vi "Main.vi"() -> ()   [LabVIEW 2017]
uses:
  type defs/action buttons.ctl
  type defs/mode buttons.ctl
  <vilib>/vision/Pattern Matching.llb/IMAQ GM Match Report.ctl
  type defs/states.ctl
  type defs/data.ctl
  <vilib>/vision/Image Controls.llb/IMAQ Image.ctl
  <vilib>/myRIO/Common/Instrument Driver Framework/myRIO v1.0/Encoder/typedefs/Encoder Signal Mode.ctl
  <vilib>/myRIO/Instrument Drivers/Onboard IO/PWM/typedefs/PWM Reference.ctl
  <vilib>/myRIO/Common/Instrument Driver Framework/Utilities/typedefs/myRIO Generic Hardware Reference.ctl
  <vilib>/myRIO/Common/Instrument Driver Framework/Utilities/typedefs/Hardware Version Enum.ctl
  <vilib>/myRIO/Common/Instrument Driver Framework/Utilities/typedefs/myRIO v1.0 Reference.ctl
  <vilib>/myRIO/Common/Instrument Driver Framework/Utilities/typedefs/Generic FPGA Reference.ctl
  <vilib>/myRIO/Common/Instrument Driver Framework/myRIO v1.0/PWM/typedefs/PWM Channels Enum.ctl
  <vilib>/myRIO/Instrument Drivers/Onboard IO/PWM/typedefs/PWM Configuration.ctl
  <vilib>/userdefined/High Color/nirio_resource_hc.ctl
  <vilib>/myRIO/Instrument Drivers/Onboard IO/DIO/typedefs/DIO Reference.ctl
  <vilib>/myRIO/Common/Instrument Driver Framework/myRIO v1.0/DIO/typedefs/DIO Channels List.ctl
  <vilib>/myRIO/Common/Instrument Driver Framework/myRIO v1.0/DIO/typedefs/DIO Channels Enum.ctl
  type defs/task.ctl
  <vilib>/myRIO/Common/Instrument Driver Framework/Utilities/vis/Is FPGA Ref Available.vi
  <vilib>/myRIO/Common/Instrument Driver Framework/myRIO v1.0/PWM/vis/myRIO v1.1 Open PWM.vi
  <vilib>/myRIO/Common/Instrument Driver Framework/myRIO v1.0/DIO/vis/myRIO v1.1 Open DIO.vi
  <vilib>/myRIO/Instrument Drivers/Onboard IO/DIO/vis/Write.vi
  <vilib>/myRIO/Common/Instrument Driver Framework/Utilities/vis/Validate Channels.vi
  <vilib>/myRIO/Common/Instrument Driver Framework/myRIO v1.0/PWM/vis/myRIO v1.0 Reserve PWM.vi
  <vilib>/myRIO/Common/Instrument Driver Framework/myRIO v1.0/DIO/vis/myRIO v1.0 Reserve DIO.vi
  <vilib>/myRIO/Common/Instrument Driver Framework/myRIO v1.0/Encoder/vis/myRIO v1.0 Close Encoder.vi
  <vilib>/myRIO/Common/Instrument Driver Framework/myRIO v1.0/PWM/vis/myRIO v1.0 Close PWM.vi
  <vilib>/myRIO/Common/Instrument Driver Framework/myRIO v1.0/UART/vis/myRIO v1.0 Close UART.vi
  <vilib>/myRIO/Common/Instrument Driver Framework/myRIO v1.0/PWM/vis/myRIO v1.0 Build MUX Configuration PWM.vi
  <vilib>/myRIO/Common/Instrument Driver Framework/myRIO v1.0/Resource Manager/vis/myRIO v1.0 Reserve Channel List.vi
  <vilib>/myRIO/Common/Instrument Driver Framework/myRIO v1.0/DIO/vis/myRIO v1.0 Build MUX Configuration DIO.vi
  <vilib>/myRIO/Common/Instrument Driver Framework/myRIO v1.0/Encoder/vis/myRIO v1.0 Unreserve Encoder.vi
  <vilib>/myRIO/Common/Instrument Driver Framework/myRIO v1.0/PWM/vis/myRIO v1.0 Unreserve PWM.vi
  <vilib>/myRIO/Common/Instrument Driver Framework/myRIO v1.0/Resource Manager/vis/myRIO v1.0 Create Configuration List.vi
  <vilib>/myRIO/Common/Instrument Driver Framework/myRIO v1.0/Resource Manager/vis/myRIO v1.0 Reserve Channel.vi
  <vilib>/myRIO/Common/Instrument Driver Framework/myRIO v1.0/Resource Manager/vis/myRIO v1.0 Unreserve Channel.vi
  <vilib>/myRIO/Common/Instrument Driver Framework/myRIO v1.0/Encoder/vis/myRIO v1.0 Build MUX Configuration Encoder.vi
  <vilib>/myRIO/Common/Instrument Driver Framework/myRIO v1.0/Resource Manager/vis/myRIO v1.0 Unreserve Channel List.vi
  <vilib>/myRIO/Common/Instrument Driver Framework/myRIO v1.0/Resource Manager/vis/myRIO v1.0 Build Mutex Name.vi
  <vilib>/Utility/VariantDataType/GetNumericInfo.vi
  <vilib>/Utility/error.llb/Error Cluster From Error Code.vi
  <vilib>/myRIO/Common/Instrument Driver Framework/myRIO v1.0/myRIO v1.1 Open.vi
  <vilib>/myRIO/Common/Instrument Driver Framework/Utilities/vis/IO Manager.vi
  <vilib>/myRIO/Common/Instrument Driver Framework/Utilities/vis/Configuration Manager.vi
  <vilib>/myRIO/Common/Instrument Driver Framework/myRIO v1.0/Resource Manager/vis/myRIO v1.0 Configure IO.vi
  <vilib>/myRIO/Common/Instrument Driver Framework/myRIO v1.0/myRIO v1.0 Close.vi
  <vilib>/myRIO/Common/Instrument Driver Framework/myRIO v1.0/Encoder/vis/myRIO v1.0 Reset Encoder.vi
  <vilib>/myRIO/Common/Instrument Driver Framework/myRIO v1.0/PWM/vis/myRIO v1.0 Write PWM.vi
  <vilib>/myRIO/Common/Instrument Driver Framework/myRIO v1.0/Encoder/vis/myRIO v1.0 Read Encoder.vi
  <vilib>/myRIO/Common/Instrument Driver Framework/myRIO v1.0/DIO/vis/myRIO v1.0 Write DIO.vi
  <vilib>/myRIO/Common/Instrument Driver Framework/myRIO v1.0/DIO/vis/myRIO v1.0 Read DIO.vi
  <vilib>/myRIO/Common/Instrument Driver Framework/myRIO v1.0/PWM/vis/myRIO v1.0 Shutdown PWM.vi
  <vilib>/myRIO/Common/Instrument Driver Framework/myRIO v1.0/Encoder/vis/myRIO v1.0 Shutdown Encoder.vi
  <vilib>/myRIO/Common/Instrument Driver Framework/Utilities/vis/FPGA Ref Manager.vi
  <vilib>/myRIO/Common/Instrument Driver Framework/myRIO v1.0/myRIO v1.0 Reset FPGA.vi
  <vilib>/myRIO/Common/Instrument Driver Framework/myRIO v1.0/IRQ/vis/myRIO v1.0 IRQ Info FGV.vi
  <vilib>/myRIO/Common/Instrument Driver Framework/myRIO v1.0/IRQ/vis/myRIO v1.0 Timer IRQ Info FGV.vi
  <vilib>/myRIO/Common/Instrument Driver Framework/myRIO v1.0/IRQ/vis/myRIO v1.0 ISR Agent.vi
  <vilib>/myRIO/Instrument Drivers/Onboard IO/I2C/typedefs/I2C Reference.ctl
  <vilib>/myRIO/Common/Instrument Driver Framework/myRIO v1.0/I2C/typedefs/I2C Channels Enum.ctl
  <vilib>/myRIO/Instrument Drivers/Onboard IO/I2C/typedefs/I2C Configuration.ctl
  <vilib>/myRIO/Instrument Drivers/Onboard IO/I2C/typedefs/I2C Transfer Rate.ctl
  <vilib>/myRIO/Express VI/Onboard IO/PWM/PWM Express VI.xnode
  <vilib>/myRIO/Instrument Drivers/Onboard IO/PWM/vis/myRIO PWM Open.xnode
  <vilib>/myRIO/Express VI/Onboard IO/DO/DO Express VI.xnode
  <vilib>/myRIO/Instrument Drivers/Onboard IO/DIO/vis/myRIO DIO Open.xnode
  <vilib>/myRIO/Express VI/Onboard Devices/LED/LED Express VI.xnode
  <vilib>/myRIO/Express VI/Onboard Devices/Button/Button Express VI.xnode
  <vilib>/myRIO/Instrument Drivers/Onboard IO/DIO/DIO.lvlib
  <vilib>/myRIO/Instrument Drivers/Onboard IO/PWM/PWM.lvlib
  <vilib>/myRIO/Instrument Drivers/Utilities/Utilities.lvlib
  <vilib>/vision/NI_Vision_Development_Module.lvlib
  <vilib>/myRIO/Instrument Drivers/Onboard IO/I2C/I2C.lvlib
  <vilib>/myRIO/Instrument Drivers/Onboard IO/I2C/vis/myRIO I2C Open.xnode
  <vilib>/myRIO/Common/Instrument Driver Framework/myRIO v1.0/I2C/vis/myRIO v1.1 Open I2C.vi
  <vilib>/myRIO/Instrument Drivers/Onboard IO/Encoder/Encoder.lvlib
panel:
  out "FT_G_enc":i32[](array[numeric])
  out "FT_M_enc":i32[](array[numeric])
  out "FT_Right_enc":i32[](array[numeric])
  out "FT_Left_enc":i32[](array[numeric])
  out "FT_Angles":dbl[](array[numeric])
  out "Dots of States":i32[][](array[numeric])
  in  "States in total":i32
  in  "(auto) States":T1(ring)
  out "R_enc_value":i32
  in  "Reset R_enc":bool
  out "L_enc_value":i32
  in  "Reset L_enc":bool
  out "G_enc":i32[](array[numeric])
  out "M_enc":i32[](array[numeric])
  out "Right_enc":i32[](array[numeric])
  out "Left_enc":i32[](array[numeric])
  out "Angles":dbl[](array[numeric])
  in  "Dots in total":i32
  in  "CurDot":T2(ring)
  out "balls to analyze":i32[](array[numeric])
  out "(auto) balls counter":i32
  out "distance to the side":u32
  out "value Z 2":ext
  out "value Z":ext
  in  ",ctl num":i32
  in  ".Task":enum16{"Def", "<mod>[P]+tnl ", "(auto)"}(ring)
  in  "_Timer":u32=1
  out "Pattern classes":i32[](array[numeric])
  in  "5":i32
  in  "4":i32
  in  "3":i32
  in  "1":i32
  in  "2":i32
  out "5":bool
  out "4":bool
  out "3":bool
  out "2":bool
  out "1":bool
  out "Color classes":i32[](array[numeric])
  in  "Next step":bool
  in  "ball = pattern?":bool
  out "error out":errorcluster
  in  "Tab Control":enum32{"Motors", "Ball", "Pattern", "Camera"}(tab)
  in  "Left+":bool
  in  "Left-":bool
  in  "Right+":bool
  in  "Right-":bool
  in  "G-":bool
  in  "G+":bool
  in  "M+":bool
  in  "M-":bool
  in  "M_PWM":dbl=0.5
  in  "L_PWM":dbl=0.5
  in  "R_PWM":dbl=0.5
  in  "Reset M_enc":bool
  out "M_enc_value":i32
  in  "Reset G_enc":bool
  out "G_enc_value":i32
  in  "G_PWM":dbl=0.5
  in  "M_UB_Align":i32=-800
  in  "G_UB_Align":i32
  in  "M_UB_grab":i32=-800
  in  "G_UB_grab":i32=-500
  in  "Manip state":enum16{"Align", "Grab", "Release"}(ring)
  in  "Balls to remember":i32
  out "Circles Calibrated (Shape Detection 1)":T3(array[cluster]) {"Position"."Y" format="%.2f"; "Position"."X" format="%.2f"}
  out "Number of Matches (Shape Detection 1)":i32
  out "Color":i32
  in  "Align X - t, Y - f":bool
  out "CircleRadius":dbl
  in  "defX":dbl=150.0
  in  "Range":dbl=40.0
  in  "defY":dbl=170.0
  out "X is in range":bool
  out "Y is in range":bool
  out "curX":dbl
  out "curY":dbl
  out "y1 (circle)":i32
  out "x1 (circle)":i32
  out "x0 (circle)":i32
  out "y0 (circle)":i32
  in  "divider (circle)":dbl=1.0
  in  "ROI Descriptor COLOR":T4={"Global Rectangle"=[86, 71, 180, 164], "Contours"=[{"ID"=enum."External", "Type"=3, "Coordinates"=[86, 71, 180, 164]}]} {"Contours"."Type" items=["No Selection", "Point", "Line", "Rectangle", "Oval", "Polygon", "Freehand Region", "Annulus", "Unused2", "Unused3", "Broken Line", "Freehand Line", "Rotated Rectangle"]}
  in  "align accuracy":u32=100
  in  "Ball number":i32=1
  out "ball match":bool
  in  "Range(p)":sgl=10.0
  in  "defX(p)":sgl=320.0
  out "Pattern":i32
  out "y0":i32
  out "x0":i32
  out "x1":i32
  out "y1":i32
  out "Number of Matches (Geometric Matching 1)":i32
  out "Calibrated Matches (Geometric Matching 1)":T5[](array[typedef]) {"Correlation Score" format="%.2f"; "Target Template Curve Score" format="%.2f"; "Template Target Curve Score" format="%.2f"; "Bounding Box"."y" format="%.2f"; "Bounding Box"."x" format="%.2f"; "Position"."y" format="%.2f"; "Position"."x" format="%.2f"; "Score" format="%.2f"; "Scale" format="%.2f"; "Angle" format="%.2f"; "Occlusion %" format="%.2f"}
  out "Scale":sgl
  in  "divider (pattern)":sgl=1.0
  out "curX(p)":sgl
  out "In Range? (p)":bool
  in  "align accuracy (p)":u32=100
  in  "pattern number":i32=1
  in  "patterns to remember":i32=3
  out "pattern match":bool
  in  "M duty cycle [P]":dbl=533.0 format="%#_13g"
  in  "S duty cycle [P]":dbl=990.0 format="%#_13g"
  in  "S duty cycle [B]":dbl=990.0 format="%#_13g"
  in  "M duty cycle [B]":dbl=533.0 format="%#_13g"
  in  "S duty cycle [F]":dbl=620.0 format="%#_13g"
  in  "M duty cycle [F]":dbl=506.0 format="%#_13g"
  in  "Angle for pattern (degrees)":sgl=90.0 format="%.2f"
  out "rotate":bool=TRUE
  in  "PWM channel (m)":tag="B/PWM2"
  in  "[cur] duty cycle [%] (m)":dbl
  in  "PWM channel (s)":tag="A/PWM2"
  in  "[cur] duty cycle [%] (s)":dbl
  in  "Camera state":enum16{"Fwd", "Pattern", "Ball"}(ring)
  in  "Angle for Align (degrees)":sgl=2.0 format="%.2f"
  in  "mode buttons":T6
  out "image display":T7(plugin-control)
  in  "action buttons":T8
  in  "Stop":bool
  # "Machine\nVision\nApp"
  # "less = slower"
  # "less = slower"
  # "0 - 640x480"
  # "5 - 1280x720"
  # "30 - 320x240"
  # "35 - 800x600"
  # "40 - 176x144"
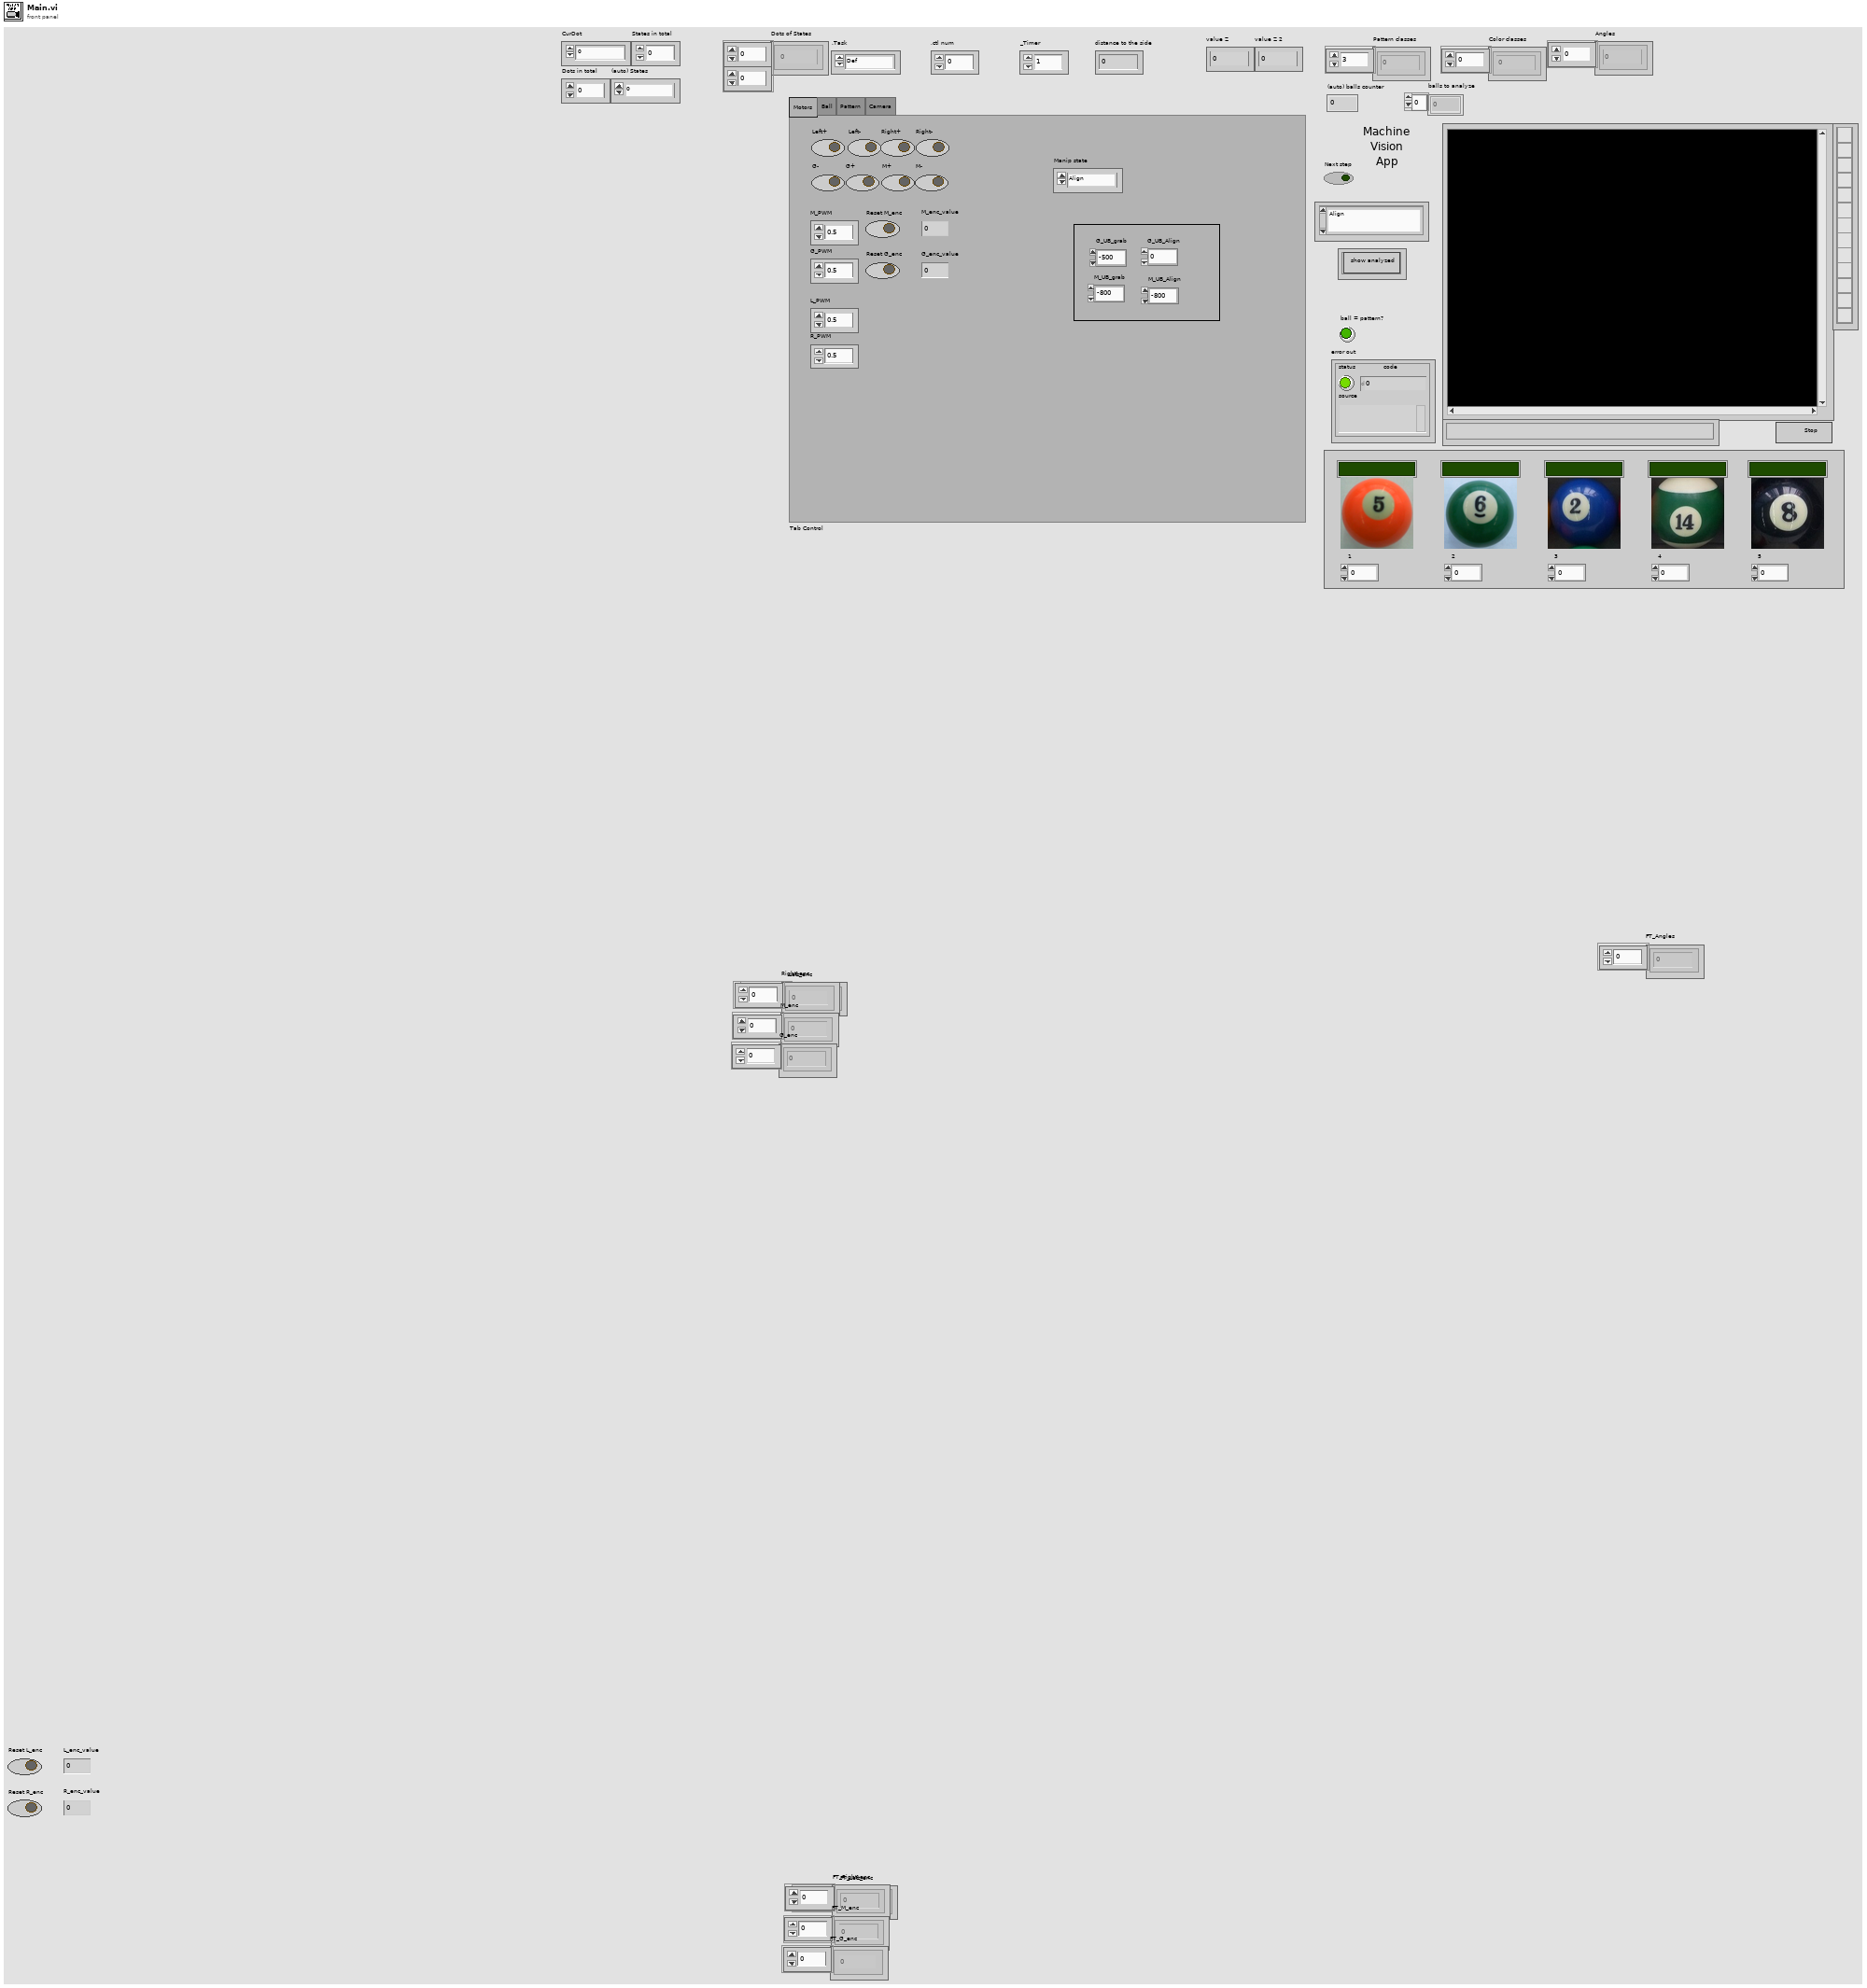
[diagram p1: front panel]
types:
  T1 = enum16{"0", "1", "2", "3", "4", "5", "6", "7", "8", "9", "10"}
  T2 = enum16{"0", "1", "2", "3", "4", "5", "6", "7", "8", "9", "10", "11", "12", "13", "14", "15", "16", "17", "18", "19", "20", "21", "22", "23", "24", "25", "26", "27", "28", "29", "30", "31", "32", "33", "34", "35"}
  T3 = cluster{"Position":cluster{"X":sgl, "Y":sgl}, "Radius":dbl, "Score":dbl}[]
  T4 = cluster{"Global Rectangle":i32[], "Contours":cluster{"ID":enum32{"External", "Internal"}, "Type":u32, "Coordinates":i32[]}[]}
  T5 = typedef "IMAQ GM Match Report.ctl" = cluster{"Position":cluster{"x":sgl, "y":sgl}, "Angle":sgl, "Scale":sgl, "Score":sgl, "Bounding Box":cluster{"x":sgl, "y":sgl}[], "Contrast Reversed":bool, "Occlusion %":sgl, "Template Target Curve Score":sgl, "Target Template Curve Score":sgl, "Correlation Score":sgl}
  T6 = typedef "mode buttons.ctl" = cluster{"show analyzed":bool}
  T7 = typedef "IMAQ Image.ctl" = refnum<image>
  T8 = typedef "action buttons.ctl" = cluster{"Shape - t, Color - f":enum16{"Align", "(pattern) Align", "Pattern", "(mod) pattern", "<mod>[P] remembering", "<mod>[P] go through tunnel", "<mod>[P] comparing", "(mod) ball", "Ball", "Other", "Clear", "navx", "(auto) Balls Analyze", "Joystick control"}}
  T9 = typedef "Encoder Signal Mode.ctl" = enum16{"Quadrature phase signal", "Step and direction signal"}
  T10 = typedef "data.ctl" = cluster{"Shape - t, Color - f":bool, "qsm":cluster{"Webcam image ref":T7, "Analyzed image ref":T7, "Stop webcam":bool}, " image ref":T7, "number img":i32, "ROI Descriptor (Image Mask 1)":cluster{"Global Rectangle":i32[], "Contours":cluster{"ID":enum32{"External", "Internal"}, "Type":u32, "Coordinates":i32[]}[]}, "Pattern class":i32, "Color class":i32, "Color classes":i32[], "Pattern classes":i32[]}
  T11 = typedef "states.ctl" = enum16{"(qsm) schedule", "(qsm) initialize", "(qsm) release", "(qsm) clean up", "(qsm) shutdown", "(myRIO) initialize", "(myRIO) clean up", "(myRIO) update ports", "Setup get", "(image) get", "(image) show", "(ball) Shape detection", "(ball) Calc ball indx", "(ball) Calculate ROI", "(ball) Analyze color", "(ball) Align", "(ball) Wait", "(ball) Grab", "(pattern) Find Square", "(pattern) Calculate ROI", "(pattern) Calc pattern indx", "Compare", "(pattern) Analyze pattern", "(pattern) Align", "(pattern) Wait", "(pattern) states control", "navx", "stop motors", "(joystick) Joystick control", "_Timer", "Setup manipulator", "(auto) Count balls", "(auto) Analyze balls", "(auto) Dot Controller", "Wait for button"}
  T12 = typedef "Encoder.lvlib/Encoder Reference.ctl" = cluster{"myRIO Reference":T13, "Encoder Channels Enum":T17}
  T13 = typedef "myRIO Generic Hardware Reference.ctl" = cluster{"myRIO Model":T14, "myRIO Hardware Reference":T15}
  T14 = typedef "Hardware Version Enum.ctl" = enum16{"Unknown", "myRIO-1900", "myRIO-1950", "roboRIO", "NI ELVIS RIO CM"}
  T15 = typedef "myRIO v1.0 Reference.ctl" = cluster{"Generic FPGA Reference":T16, "Allow multiple opens":bool}
  T16 = typedef "Generic FPGA Reference.ctl" = refnum<k20>
  T17 = typedef "Encoder Channels Enum.ctl" = enum16{"Not Connected", "C/ENC0", "C/ENC1", "A/ENC", "B/ENC", "DIO/ENC0", "DIO/ENC1", "DIO/ENC2", "DIO/ENC3", "DIO/ENC4"}
  T18 = typedef "PWM.lvlib/PWM Reference.ctl" = cluster{"myRIO Reference":T13, "PWM Channels Enum":T19, "PWM Configuration":T20}
  T19 = typedef "PWM Channels Enum.ctl" = enum16{"Not Connected", "C/PWM0", "C/PWM1", "A/PWM0", "A/PWM1", "A/PWM2", "B/PWM0", "B/PWM1", "B/PWM2", "PWM/PWM0", "PWM/PWM1", "PWM/PWM2", "PWM/PWM3", "PWM/PWM4", "PWM/PWM5", "PWM/PWM6", "PWM/PWM7", "PWM/PWM8", "PWM/PWM9"}
  T20 = typedef "PWM.lvlib/PWM Configuration.ctl" = cluster{"Frequency":dbl, "Duty Cycle":dbl}
  T21 = typedef "nirio_resource_hc.ctl" = tag
  T22 = typedef "I2C.lvlib/I2C Reference.ctl" = cluster{"myRIO Reference":T13, "I2C Channels Enum":T23, "I2C Configuration":T24}
  T23 = typedef "I2C Channels Enum.ctl" = enum16{"Not Connected", "A/I2C", "B/I2C", "I2C/I2C"}
  T24 = typedef "I2C.lvlib/I2C Configuration.ctl" = cluster{"I2C Transfer Rate":T25}
  T25 = typedef "I2C.lvlib/I2C Transfer Rate.ctl" = enum16{"Standard mode (100 kbps)", "Fast mode (400 kbps)"}
  T26 = typedef "DIO.lvlib/DIO Reference.ctl" = cluster{"myRIO Reference":T13, "DIO Channels List":T27}
  T27 = typedef "DIO Channels List.ctl" = T28[]
  T28 = typedef "DIO Channels Enum.ctl" = enum16{"Not Connected", "C/DIO0", "C/DIO1", "C/DIO2", "C/DIO3", "C/DIO4", "C/DIO5", "C/DIO6", "C/DIO7", "A/DIO0", "A/DIO1", "A/DIO2", "A/DIO3", "A/DIO4", "A/DIO5", "A/DIO6", "A/DIO7", "A/DIO8", "A/DIO9", "A/DIO10", "A/DIO11", "A/DIO12", "A/DIO13", "A/DIO14", "A/DIO15", "B/DIO0", "B/DIO1", "B/DIO2", "B/DIO3", "B/DIO4", "B/DIO5", "B/DIO6", "B/DIO7", "B/DIO8", "B/DIO9", "B/DIO10", "B/DIO11", "B/DIO12", "B/DIO13", "B/DIO14", "B/DIO15", "LED0", "LED1", "LED2", "LED3", "Button0", "DIO/DIO0", "DIO/DIO1", "DIO/DIO2", "DIO/DIO3", "DIO/DIO4", "DIO/DIO5", "DIO/DIO6", "DIO/DIO7", "DIO/DIO8", "DIO/DIO9", "SPI/CS0", "SPI/CS1", "SPI/CS2", "SPI/CS3", "LED RADIO (Green)", "LED RADIO (Red)", "LED COMM (Green)", "LED COMM (Red)", "LED MODE (Green)", "LED MODE (Red)"}
  T29 = enum16{"Align", "(pattern) Align", "Pattern", "(mod) pattern", "(mod) ball", "Ball", "Other", "Clear", "Joystick control"}
  T30 = enum16{"Align", "(pattern) Align", "Pattern", "(mod) pattern", "<mod>[P] remembering", "<mod>[P] go through tunnel", "<mod>[P] comparing", "(mod) ball", "Ball", "Other", "Clear", "navx", "(auto) Balls Analyze", "Joystick control"}
  T31 = enum16{"Align", "(pattern) Align", "Pattern", "(mod) pattern", "<mod>[P] remembering", "<mod>[P] go through tunnel", "<mod>[P] comparing", "(mod) ball", "Ball", "Other", "Clear", "Joystick control"}
  T32 = enum16{"Align", "(pattern) Align", "Pattern", "(mod) pattern", "<mod>[P]+move", "(mod) ball", "Ball", "Other", "Clear", "Joystick control"}
  T33 = typedef "task.ctl" = T11[]
  T34 = typedef "Image Type" = u32
  T35 = cluster{"Position":cluster{"X":sgl, "Y":sgl}, "Radius":dbl, "Score":dbl}
  T36 = cluster{"ID":enum32{"External", "Internal"}, "Type":u32, "Coordinates":i32[]}[]
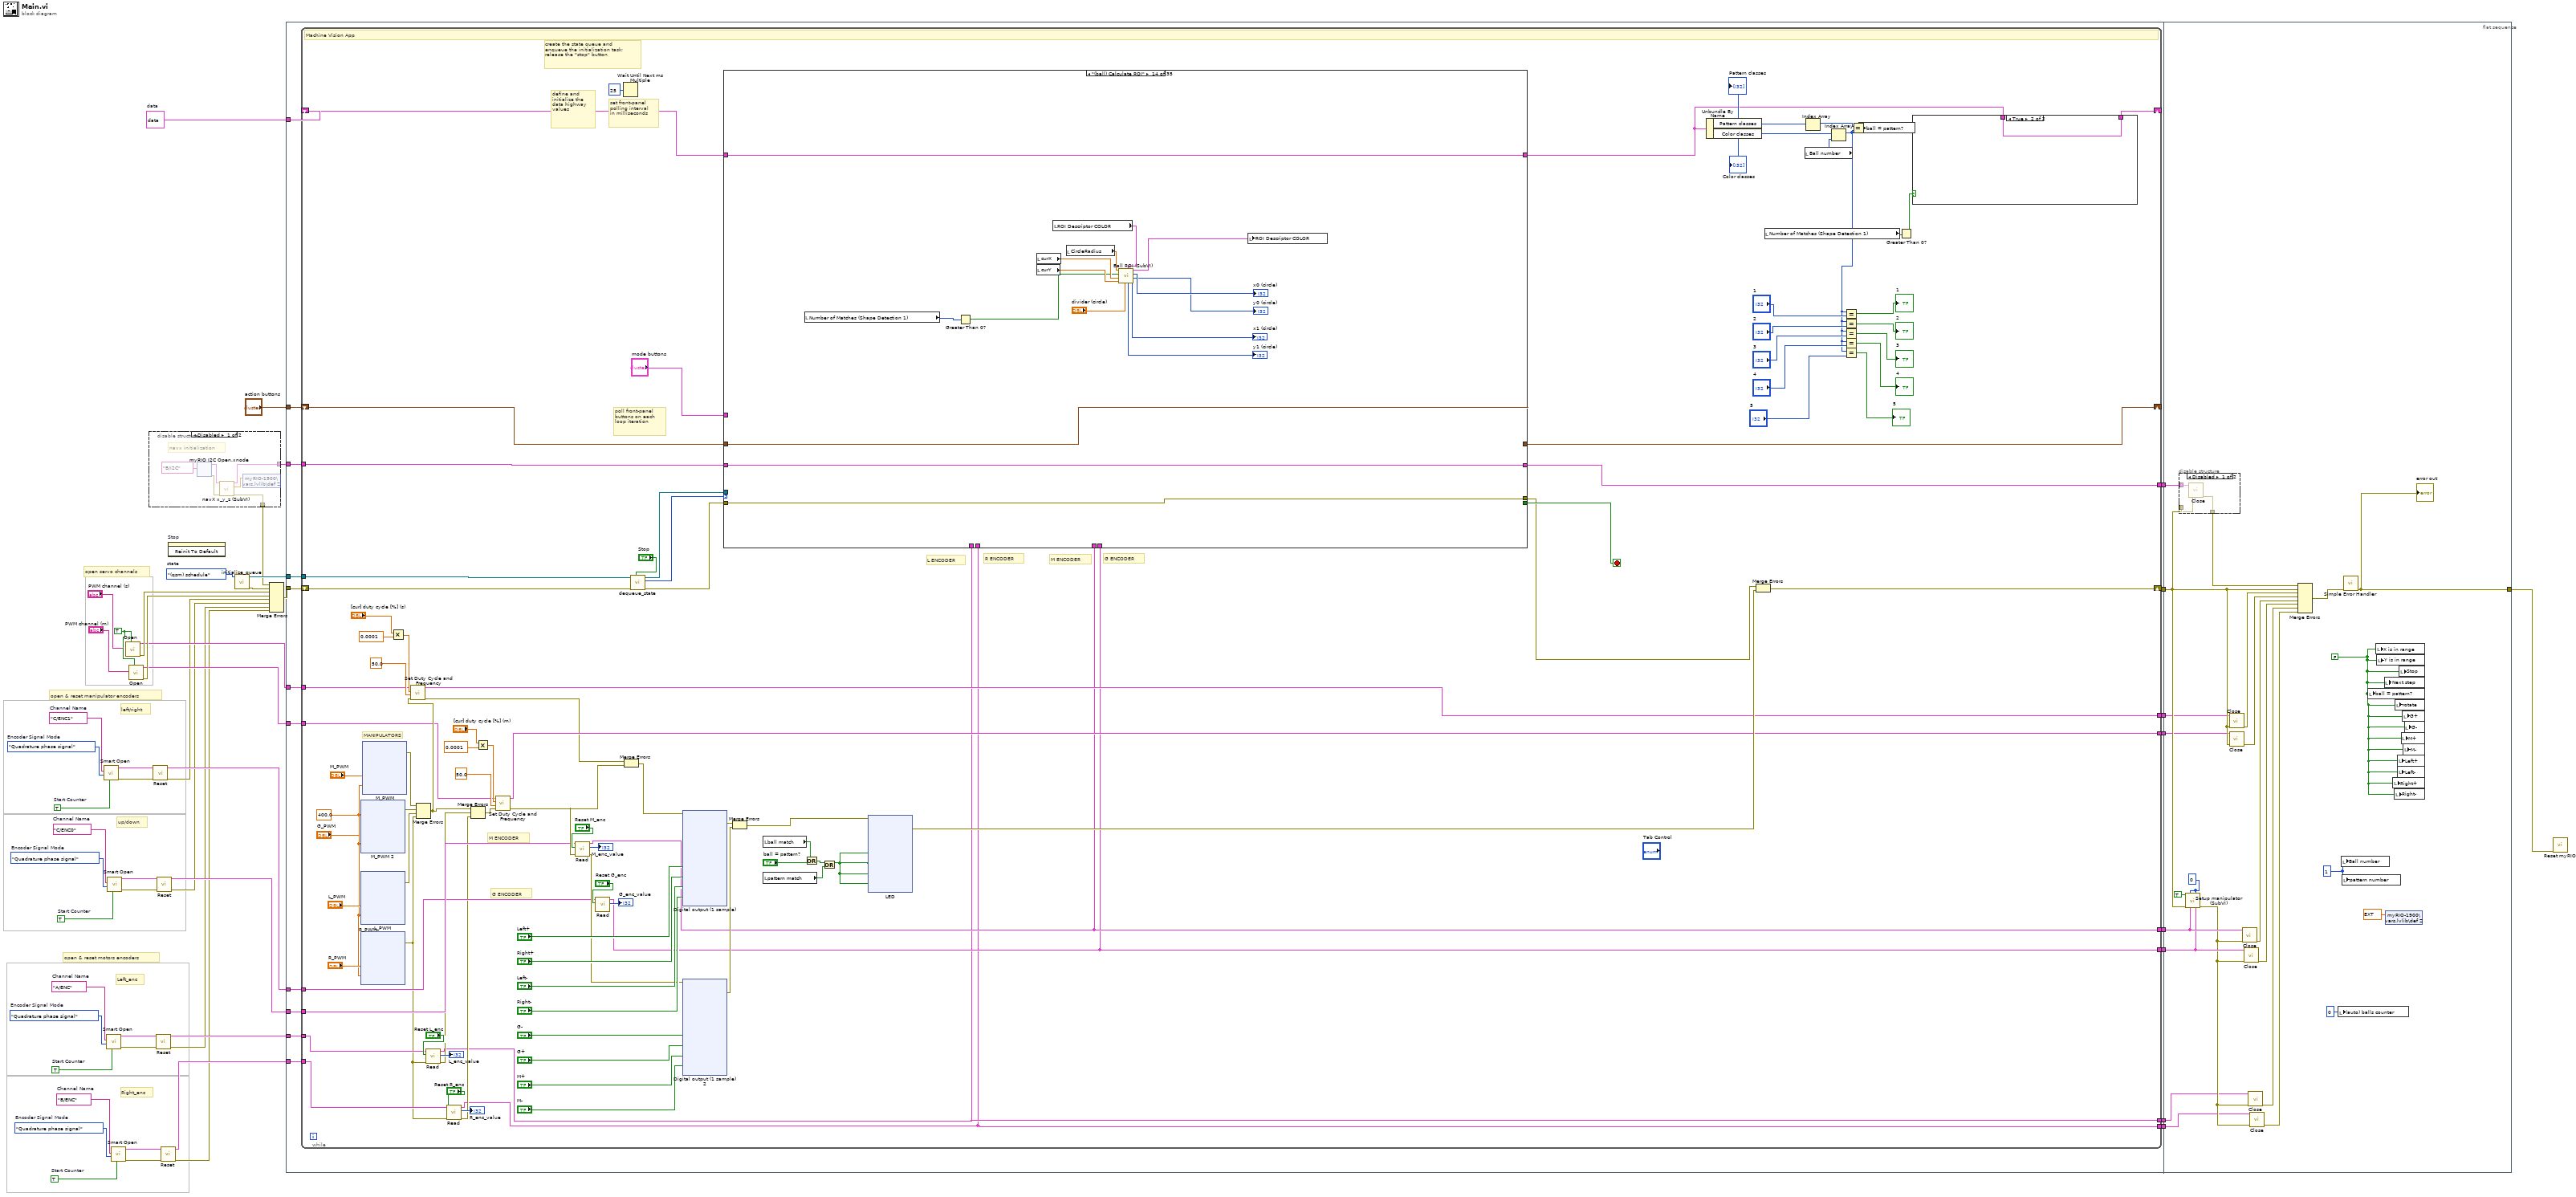
[diagram p0: block diagram]
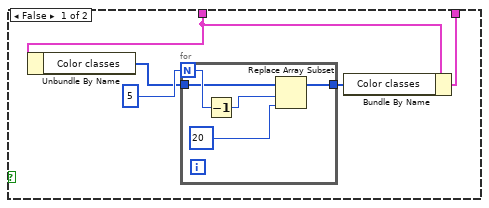
[diagram p3: hidden frame]
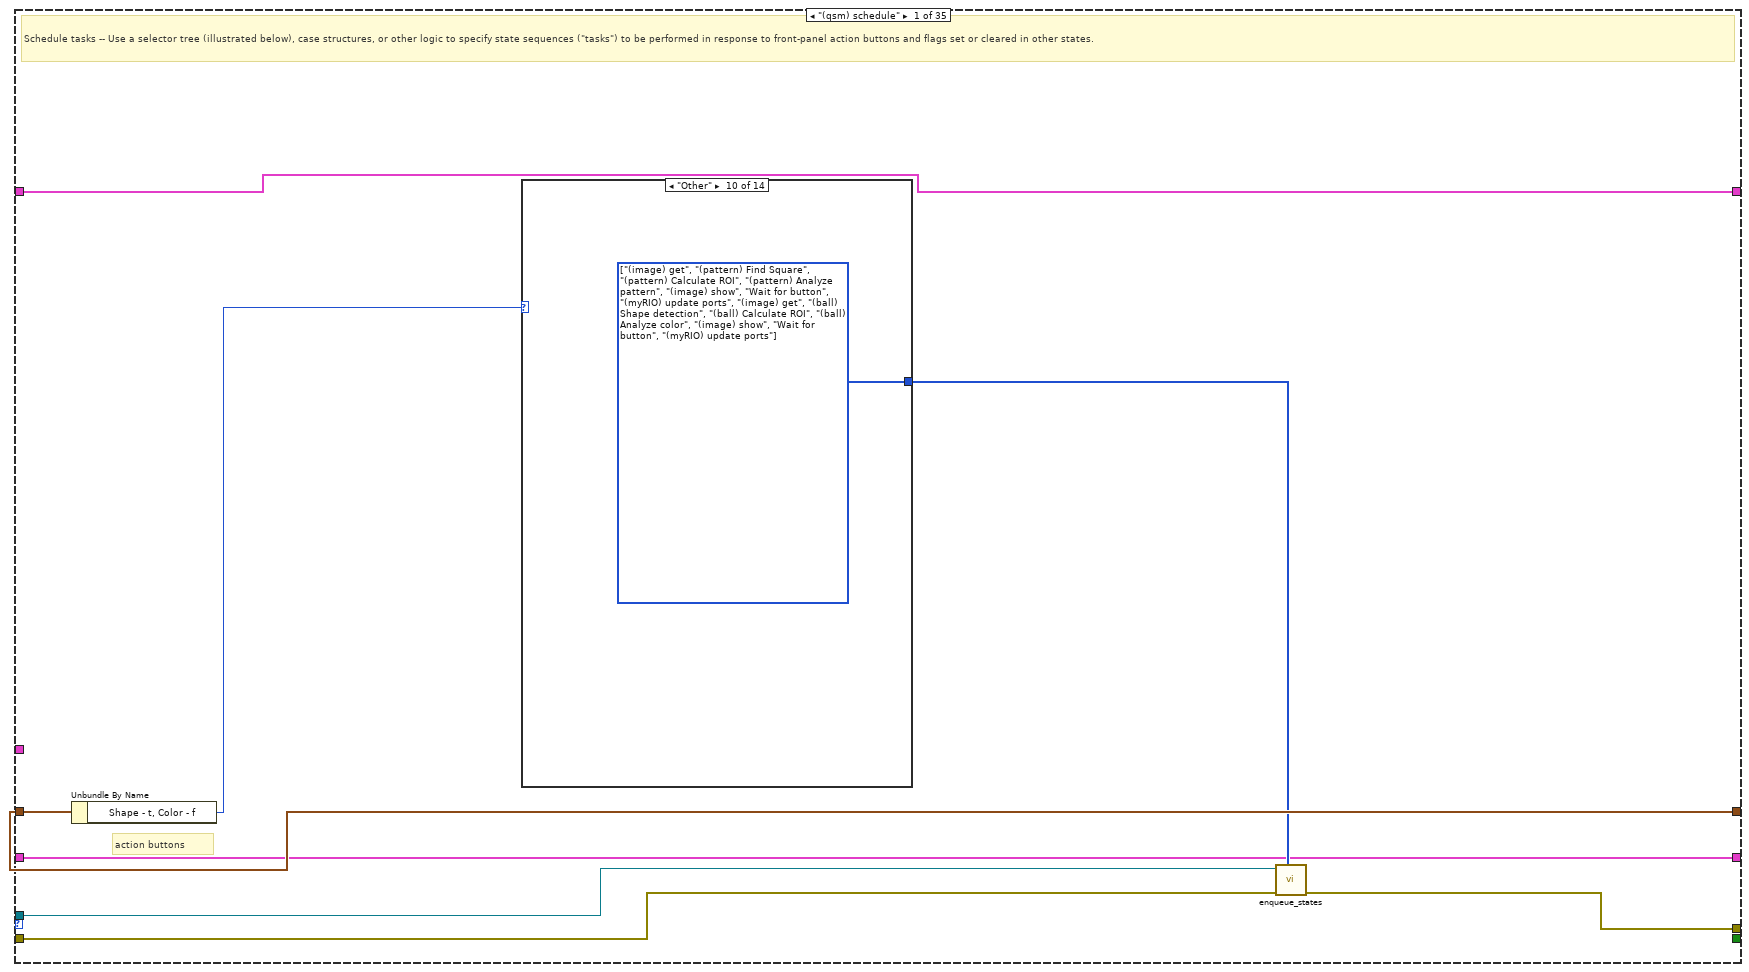
[diagram p4: hidden frame]
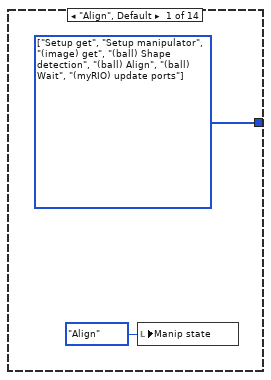
[diagram p5: hidden frame]
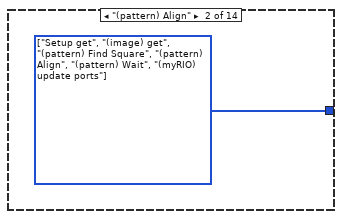
[diagram p6: hidden frame]
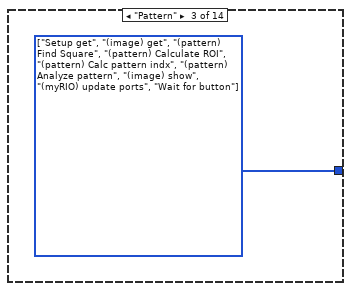
[diagram p7: hidden frame]
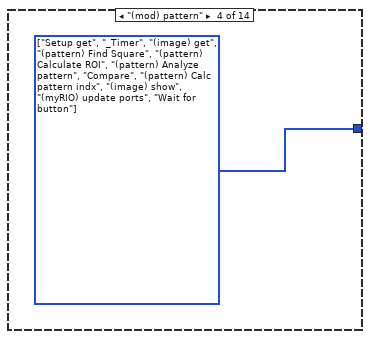
[diagram p8: hidden frame]
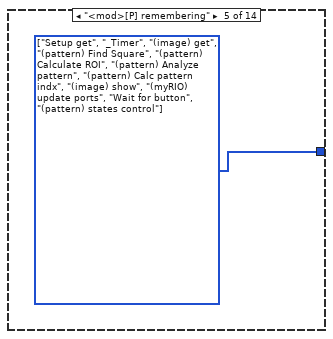
[diagram p9: hidden frame]
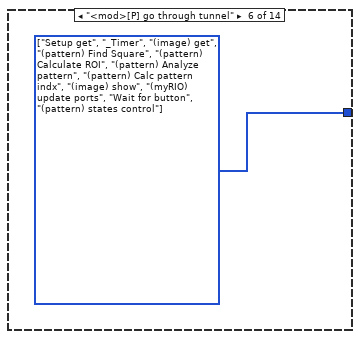
[diagram p10: hidden frame]
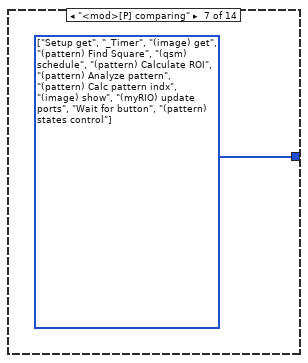
[diagram p11: hidden frame]
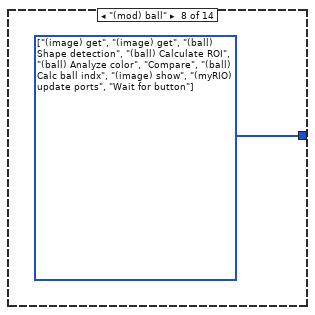
[diagram p12: hidden frame]
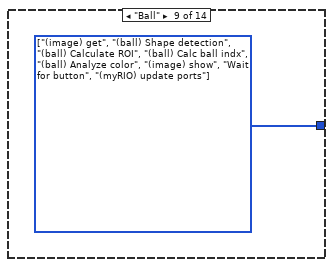
[diagram p13: hidden frame]
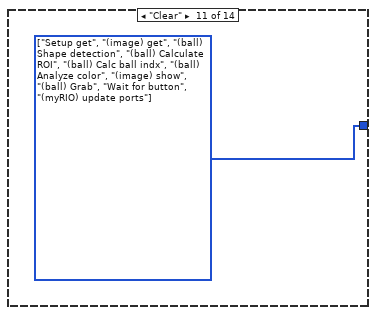
[diagram p14: hidden frame]
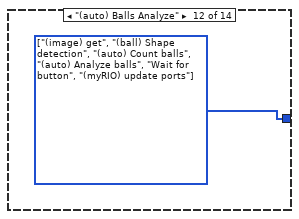
[diagram p15: hidden frame]
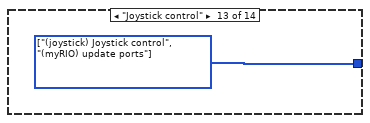
[diagram p16: hidden frame]
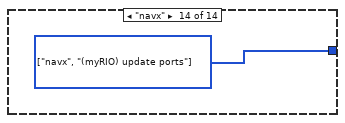
[diagram p17: hidden frame]
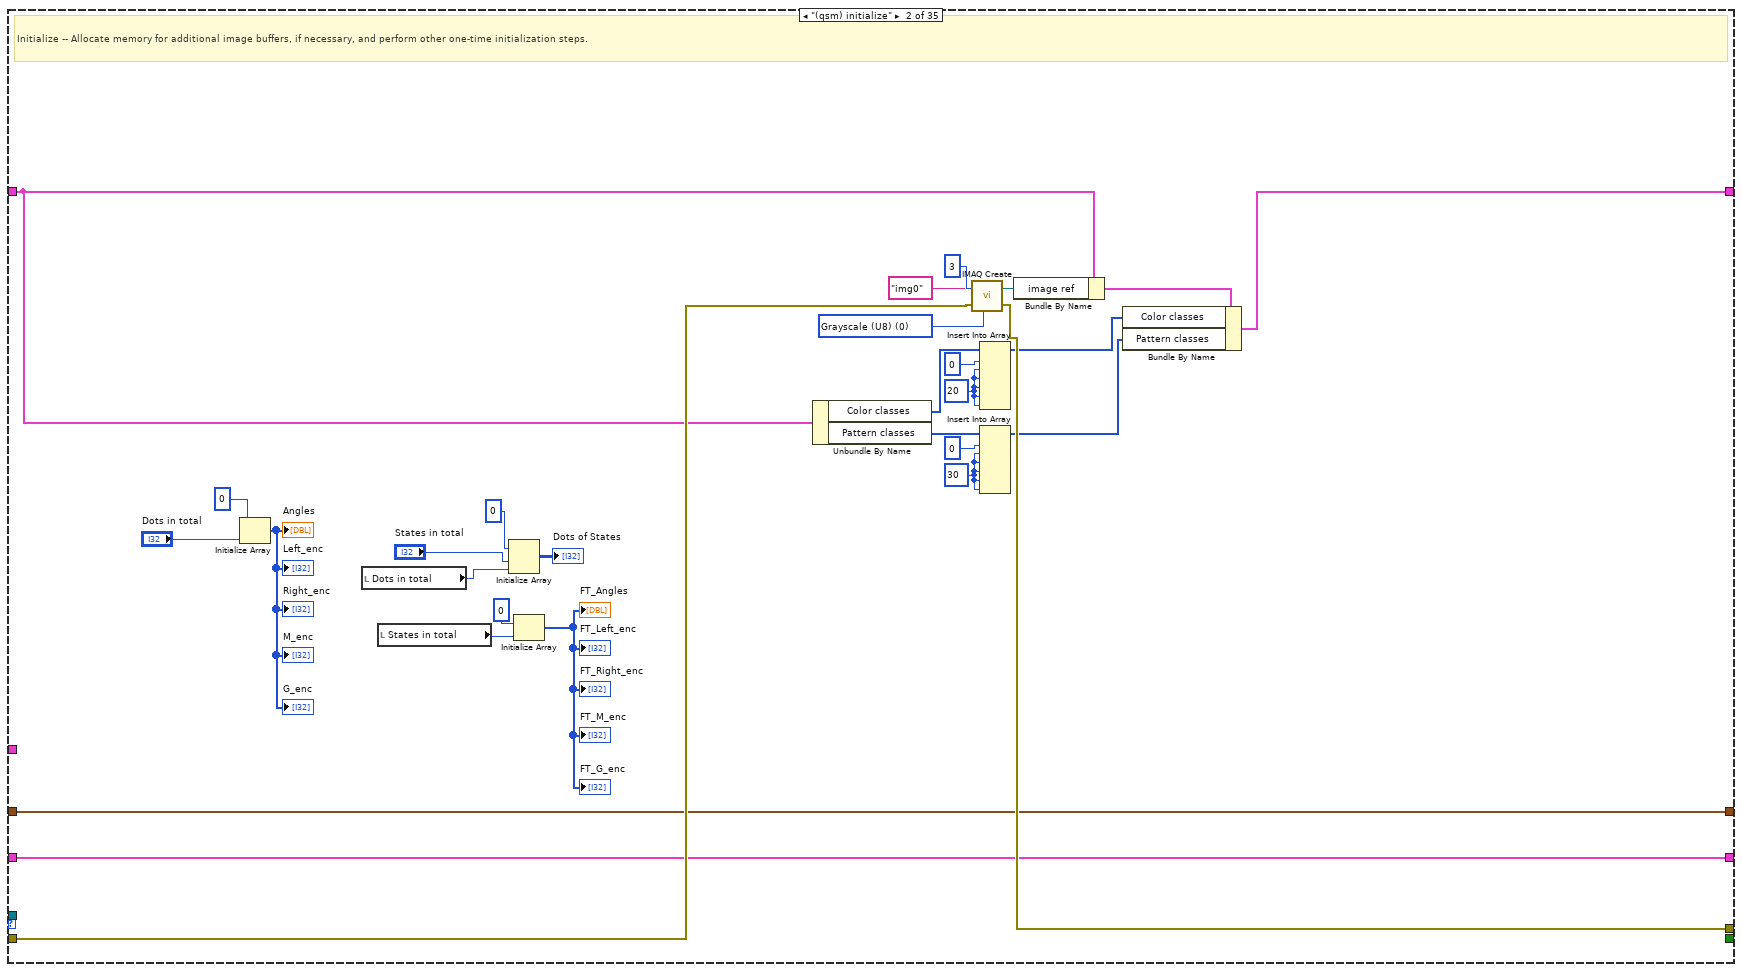
[diagram p18: hidden frame]
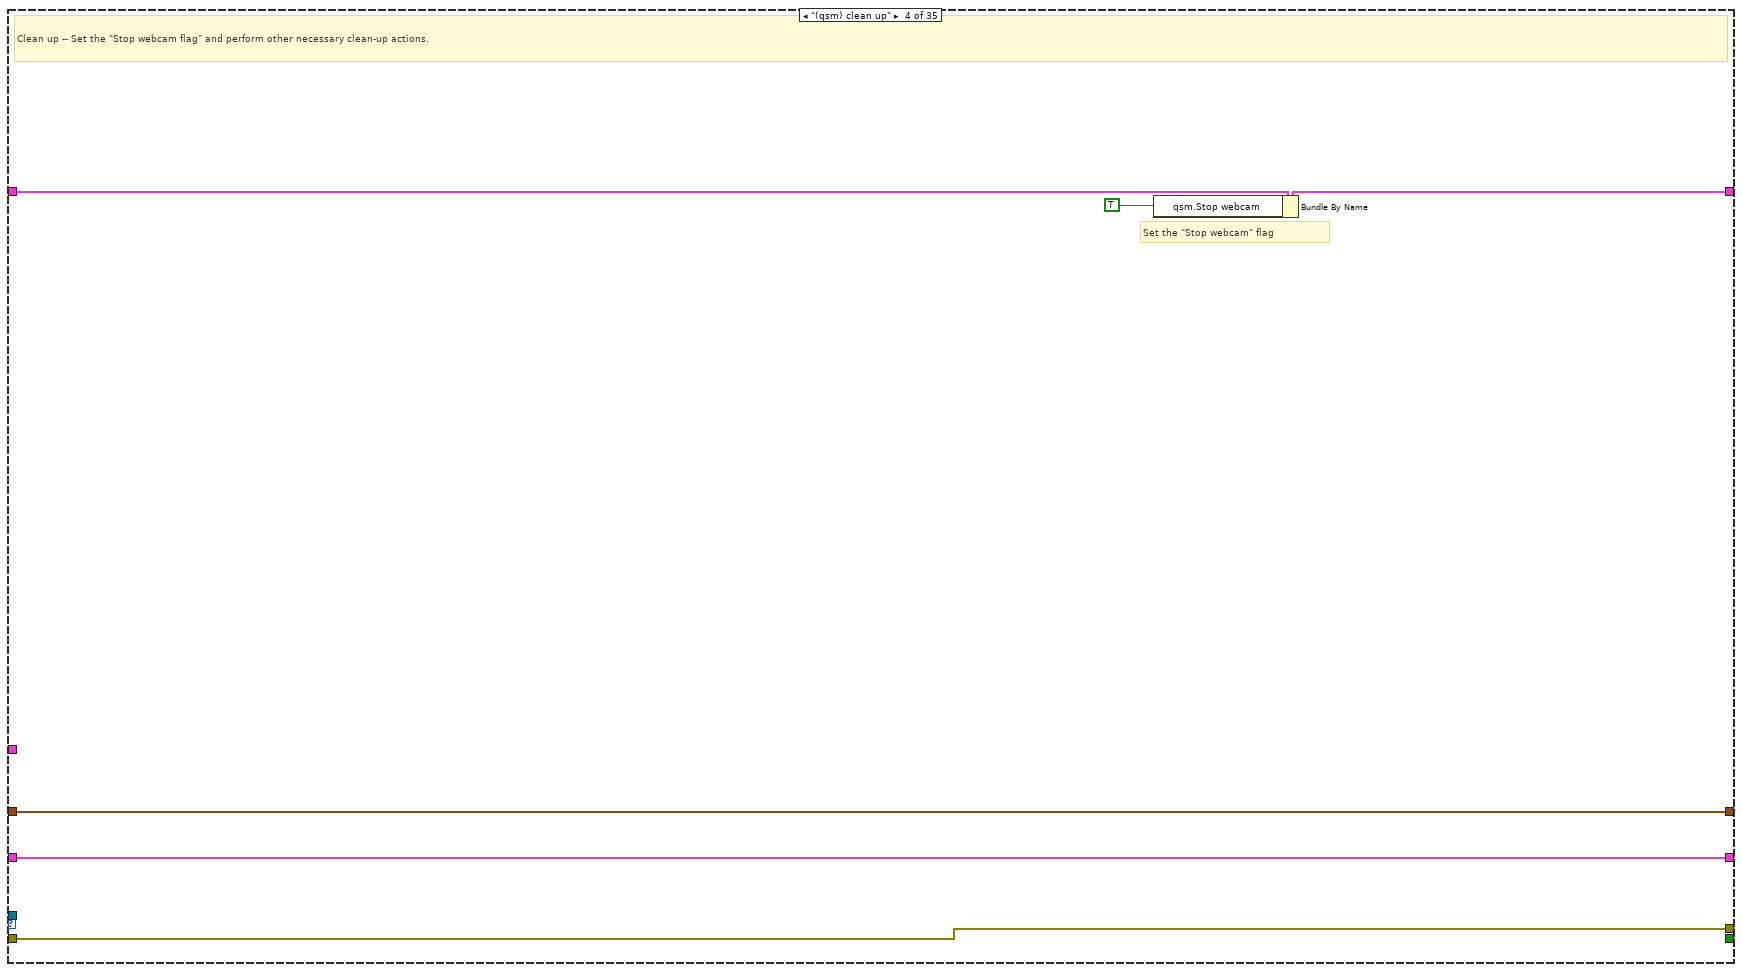
[diagram p20: hidden frame]
diagram:
  w8 = TRUE  # Start Counter
  w7 = TRUE  # Start Counter
  w11 = Encoder_Signal_Mode."Quadrature phase signal"  # Encoder Signal Mode
  w12 = tag "B/ENC"  # Channel Name
  w15 = Encoder_Signal_Mode."Quadrature phase signal"  # Encoder Signal Mode
  w16 = tag "A/ENC"  # Channel Name
  w24 = TRUE  # Start Counter
  w25 = Encoder_Signal_Mode."Quadrature phase signal"  # Encoder Signal Mode
  w26 = tag "C/ENC1"  # Channel Name
  w30 = TRUE  # Start Counter
  w31 = Encoder_Signal_Mode."Quadrature phase signal"  # Encoder Signal Mode
  w32 = tag "C/ENC0"  # Channel Name
  w39 = TRUE ("Allow multiple opens?")
  w36 = T10 {"Shape - t, Color - f"=FALSE, "qsm"={"Webcam image ref"=refnum, "Analyzed image ref"=refnum, "Stop webcam"=FALSE}, " image ref"=refnum, "number img"=0, "ROI Descriptor (Image Mask 1)"={"Global Rectangle"=[109, 72, 345, 284], "Contours"=[{"ID"=enum."External", "Type"=3, "Coordinates"=[109, 72, 345, 284]}]}, "Pattern class"=0, "Color class"=0, "Color classes"=[], "Pattern classes"=[]}  # data
  w47 = states."(qsm) schedule"  # state
  # "open & reset motors encoders"
  # "Right_enc"
  # "Left_enc"
  # "left/right"
  # "up/down"
  # "open servo channels"
  # "open & reset manipulator encoders"
  n1 = call <vilib>:"Smart Open.vi"("Start Counter"=w24, "Encoder Signal Mode"=w25, "Channel Name"=w26) -> ("error out"=w22:errorcluster, "Encoder Ref Out"=w23:T12)  [unwired: 7 in]
  n2 = call <vilib>:"Smart Open.vi"("Start Counter"=w7, "Encoder Signal Mode"=w15, "Channel Name"=w16) -> ("error out"=w13:errorcluster, "Encoder Ref Out"=w14:T12)  [unwired: 7 in]
  n3 = call <vilib>:"Smart Open.vi"("Start Counter"=w30, "Encoder Signal Mode"=w31, "Channel Name"=w32) -> ("error out"=w28:errorcluster, "Encoder Ref Out"=w29:T12)  [unwired: 7 in]
  n4 = call <vilib>:"Smart Open.vi"("Start Counter"=w8, "Encoder Signal Mode"=w11, "Channel Name"=w12) -> ("error out"=w9:errorcluster, "Encoder Ref Out"=w10:T12)  [unwired: 7 in]
  n5 = call <vilib>:"Open.vi"("Allow multiple opens?"=w39, "Channel Name"="PWM channel (s)") -> ("error out"=w45:errorcluster, "PWM Ref Out"=w43:T18)  [unwired: 8 in]
  n6 = call <vilib>:"Open.vi"("Allow multiple opens?"=w39, "Channel Name"="PWM channel (m)") -> ("error out"=w44:errorcluster, "PWM Ref Out"=w42:T18)  [unwired: 8 in]
  n7 = disable-structure shown="Disabled" {
    disable-tunnel: [w56 _] -> w34
    disable-tunnel: [w54 _] -> w33
    frame Disabled {
      # "navx initialization"
      n8 = xnode "myRIO I2C Open.xnode"("Channel Name"=tag "B/I2C") -> ("error out"=w53:errorcluster, "I2C Ref Out"=w55:T22)  [unwired: 2 in]
      n9 = call "navX x_y_z (SubVI).vi"("I2C Ref Out in"=w55, "error in (no error)"=w53) -> ("I2C Ref Out out"=w54:T22, "value Z"=w57:ext, "error out"=w56:errorcluster)  [unwired: 9 in, 2 out]
      n10 = shared-variable "myRIO-1900\\vars.lvlib\\def Z"(w57) -> ()  [unwired: 1 in, 1 out]
    }
    frame Enabled {
    }
  }
  n11 = call <vilib>:"Reset.vi"("error in (no error)"=w22, "Encoder Ref In"=w23) -> ("error out"=w17:errorcluster, "Encoder Ref Out"=w21:T12)  [unwired: 8 in]
  n12 = call <vilib>:"Reset.vi"("error in (no error)"=w13, "Encoder Ref In"=w14) -> ("error out"=w4:errorcluster, "Encoder Ref Out"=w6:T12)  [unwired: 8 in]
  n13 = call <vilib>:"Reset.vi"("error in (no error)"=w28, "Encoder Ref In"=w29) -> ("error out"=w18:errorcluster, "Encoder Ref Out"=w27:T12)  [unwired: 8 in]
  n14 = call <vilib>:"Reset.vi"("error in (no error)"=w9, "Encoder Ref In"=w10) -> ("error out"=w3:errorcluster, "Encoder Ref Out"=w5:T12)  [unwired: 8 in]
  n15 = invoke on="Stop" class="Bool (strict)" method="Reinit To Default"() -> ()  [unwired: 3 in, 3 out]
  n16 = call "initialize_queue.vi"("state"=w47) -> ("error out"=w48:errorcluster, "queue out"=w49:refnum<queue>)  [unwired: 9 in]
  n17 = Merge Errors(w34, w48, w45, w44, w17, w18, w4, w3) -> (w46:errorcluster)
  n18 = flat-sequence {
    tunnel: [w93] -> w51
    tunnel: "action buttons" -> [w92]
    tunnel: w46 -> [w90]
    tunnel: w49 -> [w91]
    tunnel: w36 -> [w89]
    tunnel: w43 -> [w88]
    tunnel: w42 -> [w87]
    tunnel: [w86] -> w41
    tunnel: [w85] -> w40
    tunnel: w33 -> [w84]
    tunnel: [w83] -> w35
    tunnel: w27 -> [w82]
    tunnel: w21 -> [w81]
    tunnel: [w80] -> w20
    tunnel: [w79] -> w19
    tunnel: w6 -> [w78]
    tunnel: w5 -> [w77]
    tunnel: [w76] -> w2
    tunnel: [w75] -> w1
    tunnel: [w1249] -> w52
    tunnel: w51 -> [w1238]
    tunnel: w41 -> [w1236]
    tunnel: w40 -> [w1235]
    tunnel: w35 -> [w1244]
    tunnel: w20 -> [w1233]
    tunnel: w19 -> [w1234]
    tunnel: w2 -> [w1228]
    tunnel: w1 -> [w1229]
    frame #0 {
      n19 = while {
        shift-right: [w185] -> w93
        shift-left: w90 -> [w190]
        shift-right: [w164] -> _
        shift-left: w89 -> [w158]
        shift-right: [w174] -> _
        shift-left: w92 -> [w173]
        tunnel: w91 -> [w172]
        tunnel: w88 -> [w132]
        tunnel: w87 -> [w116]
        tunnel: [w129] -> w86
        tunnel: [w128] -> w85
        tunnel: w84 -> [w126]
        tunnel: [w125] -> w83
        tunnel: w82 -> [w118]
        tunnel: w81 -> [w117]
        tunnel: [w114] -> w80
        tunnel: [w115] -> w79
        tunnel: w78 -> [w101]
        tunnel: w77 -> [w100]
        tunnel: [w95] -> w76
        tunnel: [w94] -> w75
        stop <- w171 stop-if-true
        w107 = 400.0 ("Frequency [Hz]")
        # "R ENCODER"
        # "L ENCODER"
        # "G ENCODER"
        # "M ENCODER"
        # "G ENCODER"
        # "M ENCODER"
        # "define and \ninitialize the \ndata highway\nvalues"
        # "MANIPULATORS"
        # "create the state queue and\nenqueue the initialization task;\nrelease the \"stop\" button"
        # "set front-panel\npolling interval\nin milliseconds"
        # "poll front-panel\nbuttons on each\nloop iteration"
        # "Machine Vision App"
        n20 = xnode "M_PWM 2"("Duty Cycle"="G_PWM", "Frequency [Hz]"=w107) -> ("error out"=w108:errorcluster)  [unwired: 1 in]
        n21 = xnode "L_PWM"("Duty Cycle"="L_PWM", "Frequency [Hz]"=w107) -> ("error out"=w184:errorcluster)  [unwired: 1 in]
        n22 = xnode "R_PWM"("Duty Cycle"="R_PWM", "Frequency [Hz]"=w107) -> ("error out"=w99:errorcluster)  [unwired: 1 in]
        n23 = xnode "M_PWM"("Duty Cycle"="M_PWM", "Frequency [Hz]"=w107) -> ("error out"=w109:errorcluster)  [unwired: 1 in]
        n24 = Multiply(x="[cur] duty cycle [%] (s)", y=0.0001) -> (x*y=w135:dbl)
        n25 = Merge Errors(w109, w108, w184, w99) -> (w131:errorcluster)
        n26 = call <vilib>:"Set Duty Cycle and Frequency.vi"("error in (no error)"=w131, "Frequency [Hz]"=50.0 ("freq [Hz]"), "Duty Cycle"=w135, "PWM Ref In"=w132) -> ("error out"=w127:errorcluster, "PWM Ref Out"=w129:T18)  [unwired: 5 in]
        n27 = call <vilib>:"Read.vi"("error in (no error)"=w99, "Reset Counter"="Reset L_enc", "Encoder Ref In"=w101) -> ("error out"=w97:errorcluster, "Counter Value"=→"L_enc_value":i32, "Encoder Ref Out"=w95:T12)  [unwired: 4 in, 2 out]
        n28 = call <vilib>:"Read.vi"("error in (no error)"=w99, "Reset Counter"="Reset R_enc", "Encoder Ref In"=w100) -> ("error out"=w96:errorcluster, "Counter Value"=→"R_enc_value":i32, "Encoder Ref Out"=w94:T12)  [unwired: 4 in, 2 out]
        n29 = Merge Errors(w131, w97, w96) -> (w98:errorcluster)
        n30 = Multiply(x="[cur] duty cycle [%] (m)", y=0.0001) -> (x*y=w139:dbl)
        n31 = call <vilib>:"Set Duty Cycle and Frequency.vi"("error in (no error)"=w98, "Frequency [Hz]"=50.0 ("freq [Hz]"), "Duty Cycle"=w139, "PWM Ref In"=w116) -> ("error out"=w122:errorcluster, "PWM Ref Out"=w128:T18)  [unwired: 5 in]
        n32 = call <vilib>:"Read.vi"("error in (no error)"=w122, "Reset Counter"="Reset M_enc", "Encoder Ref In"=w118) -> ("error out"=w121:errorcluster, "Counter Value"=→"M_enc_value":i32, "Encoder Ref Out"=w115:T12)  [unwired: 4 in, 2 out]
        n33 = call <vilib>:"Read.vi"("Reset Counter"="Reset G_enc", "Encoder Ref In"=w117) -> ("Counter Value"=→"G_enc_value":i32, "Encoder Ref Out"=w114:T12)  [unwired: 5 in, 3 out]
        n34 = Wait Until Next ms Multiple(millisecond multiple=u32 25) -> ()  [unwired: 1 out]
        n35 = Merge Errors(w127, w122) -> (w130:errorcluster)
        n36 = call "dequeue_state.vi"("stop"="Stop", "error in (no error)"=w190, "queue in"=w172) -> ("error out"=w191:errorcluster, "state"=w186:T11, "queue out"=w175:refnum<queue>)  [unwired: 6 in]
        n37 = xnode "Digital output (1 sample)"("Left+ (A/DIO5 (Pin 21))"="Left+", "Right+ (A/DIO7 (Pin 25))"="Right+", "Left- (A/DIO6 (Pin 23))"="Left-", "Right- (A/DIO13 (Pin 26))"="Right-", "error in (no error)"=w130) -> ("error out"=w183:errorcluster)
        n38 = xnode "Digital output (1 sample) 2"("G- (B/DIO7 (Pin 25))"="G-", "G+ (B/DIO13 (Pin 26))"="G+", "M+ (B/DIO5 (Pin 21))"="M+", "M- (B/DIO6 (Pin 23))"="M-", "error in (no error)"=w121) -> ("error out"=w182:errorcluster)
        n39 = case shown="\"(ball) Calculate ROI\"" w186 {
          tunnel: w191 -> [w461 w508 w511 w515 w527 w530 w535 w581 w667 w691 w713 w735 w741 w768 w772 w787 w812 w841 w859 w879 w884 w894 w937 w947 w954 w971 w1018 w1046 w1058 w1067 w1076 w1090 w1097 w1137 w1184]
          tunnel: w175 -> [w462 _ _ _ w526 _ _ _ _ _ _ _ _ _ _ _ w810 _ _ _ _ _ _ _ _ _ _ _ _ _ _ _ w1098 w1132 _]
          tunnel: [w463 w507 w511 w515 w522 w530 w534 w579 w667 w684 w713 w730 w741 w768 w771 w787 w811 w840 w860 w879 w884 w894 w936 w947 w954 w971 w1027 w1046 w1058 w1067 w1075 w1090 w1096 w1130 w1184] -> w161
          tunnel: w173 -> [w460 w502 w510 w514 w521 w529 w533 w577 w668 w683 w710 w727 w740 w766 w781 w786 w814 w834 w848 w877 w885 w892 w932 w948 w951 w970 w1029 w1048 w1063 w1068 w1074 w1092 w1100 w1139 w1185]
          tunnel: w158 -> [w464 w499 w512 w517 w525 w531 w537 w582 w669 w693 w714 w732 w742 w767 w784 w788 w816 w843 w844 w878 w886 w893 w935 w949 w955 w972 w1030 w1049 w1064 w1069 w1080 w1093 w1101 w1140 w1182]
          tunnel: [w464 w500 w512 w516 w525 w531 w537 w582 w669 w694 w714 w731 w742 w767 w783 w788 w815 w843 w858 w866 w886 w893 w934 w949 w955 w972 w1030 w1049 w1064 w1069 w1080 w1093 w1101 w1140 w1182] -> w165
          tunnel: "mode buttons" -> [_ _ _ _ _ _ _ _ _ _ w712 _ _ _ _ _ _ _ _ _ _ _ _ _ _ _ _ _ _ _ _ _ _ _ _]
          tunnel: [w460 w502 w510 w514 w521 w529 w533 w577 w668 w683 w710 w727 w740 w766 w781 w786 w813 w833 w850 w877 w885 w892 w932 w948 w953 w969 w1029 w1048 w1063 w1068 w1074 w1092 w1100 w1139 w1185] -> w174
          tunnel: [_ _ _ _ TRUE _ _ _ _ _ _ _ _ _ _ _ _ _ _ _ _ _ _ _ _ _ w1016 _ _ _ _ _ _ _ _] -> w171
          tunnel: w126 -> [w457 w490 w509 w513 w519 w528 w532 w576 w666 w688 w709 w718 w736 w754 w769 w785 w809 w842 w845 w865 w881 w887 w926 w940 w950 w968 w1023 w1047 w1052 w1065 w1079 w1091 w1099 w1138 w1181]
          tunnel: [w457 w490 w509 w513 w519 w528 w532 w576 w666 w688 w709 w718 w736 w754 w769 w785 w809 w842 w845 w865 w881 w887 w926 w940 w950 w968 w1028 w1047 w1052 w1065 w1079 w1091 w1099 w1126 w1181] -> w125
          tunnel: w115 -> [_ _ _ _ _ _ _ _ _ _ _ _ _ _ _ _ _ w839 _ _ _ _ _ _ _ _ _ _ _ _ w1078 _ _ w1134 _]
          tunnel: w114 -> [_ _ _ _ _ _ _ _ _ _ _ _ _ _ _ _ _ w838 _ _ _ _ _ _ _ _ _ _ _ _ w1077 _ _ w1133 _]
          tunnel: w95 -> [_ _ _ _ _ _ _ _ _ _ _ _ _ _ _ _ _ _ _ _ _ _ _ _ _ _ _ _ _ _ _ _ _ w1136 _]
          tunnel: w94 -> [_ _ _ _ _ _ _ _ _ _ _ _ _ _ _ _ _ _ _ _ _ _ _ _ _ _ _ _ _ _ _ _ _ w1135 _]
          frame "(qsm) schedule" {
            # "action buttons"
            # "Schedule tasks -- Use a selector tree (illustrated below), case structures, or other logic to specify state sequences (\"tasks\") to be performed in response to front-panel action buttons and flags set or cleared in other states."
            n40 = Unbundle By Name(w460) -> ("Shape - t, Color - f"=w459:T30)
            n41 = case shown="\"Other\"" w459 {
              tunnel: [w466 w467 w468 w469 w470 w471 w472 w473 w474 w475 w476 w477 w478 w479] -> w458
              frame "Align", Default {
                w466 = T33 [enum."Setup get", enum."Setup manipulator", enum."(image) get", enum."(ball) Shape detection", enum."(ball) Align", enum."(ball) Wait", enum."(myRIO) update ports"] items=["(qsm) schedule", "(qsm) initialize", "(qsm) release", "(qsm) clean up", "(qsm) shutdown", "(myRIO) initialize", "(myRIO) clean up", "(myRIO) update ports", "Setup get", "(image) get", "(image) show", "(ball) Shape detection", "(ball) Calc ball indx", "(ball) Calculate ROI", "(ball) Analyze color", "(ball) Align", "(ball) Wait", "(ball) Grab", "(pattern) Find Square", "(pattern) Calculate ROI", "(pattern) Calc pattern indx", "Compare", "(pattern) Analyze pattern", "(pattern) Align", "(pattern) Wait", "(pattern) states control", "navx", "stop motors", "(joystick) Joystick control", "_Timer", "Setup manipulator", "(auto) Count balls", "(auto) Analyze balls", "(auto) Dot Controller", "Wait for button"]
                n42 = local write "Manip state"(enum16{"Align", "Grab", "Release"}."Align" ("Manip state")) -> ()
              }
              frame "(pattern) Align" {
                w467 = T33 [enum."Setup get", enum."(image) get", enum."(pattern) Find Square", enum."(pattern) Align", enum."(pattern) Wait", enum."(myRIO) update ports"] items=["(qsm) schedule", "(qsm) initialize", "(qsm) release", "(qsm) clean up", "(qsm) shutdown", "(myRIO) initialize", "(myRIO) clean up", "(myRIO) update ports", "Setup get", "(image) get", "(image) show", "(ball) Shape detection", "(ball) Calc ball indx", "(ball) Calculate ROI", "(ball) Analyze color", "(ball) Align", "(ball) Wait", "(ball) Grab", "(pattern) Find Square", "(pattern) Calculate ROI", "(pattern) Calc pattern indx", "Compare", "(pattern) Analyze pattern", "(pattern) Align", "(pattern) Wait", "(pattern) states control", "navx", "stop motors", "(joystick) Joystick control", "_Timer", "Setup manipulator", "(auto) Count balls", "(auto) Analyze balls", "(auto) Dot Controller", "Wait for button"] ("task")
              }
              frame "Pattern" {
                w468 = T33 [enum."Setup get", enum."(image) get", enum."(pattern) Find Square", enum."(pattern) Calculate ROI", enum."(pattern) Calc pattern indx", enum."(pattern) Analyze pattern", enum."(image) show", enum."(myRIO) update ports", enum."Wait for button"] items=["(qsm) schedule", "(qsm) initialize", "(qsm) release", "(qsm) clean up", "(qsm) shutdown", "(myRIO) initialize", "(myRIO) clean up", "(myRIO) update ports", "Setup get", "(image) get", "(image) show", "(ball) Shape detection", "(ball) Calc ball indx", "(ball) Calculate ROI", "(ball) Analyze color", "(ball) Align", "(ball) Wait", "(ball) Grab", "(pattern) Find Square", "(pattern) Calculate ROI", "(pattern) Calc pattern indx", "Compare", "(pattern) Analyze pattern", "(pattern) Align", "(pattern) Wait", "(pattern) states control", "navx", "stop motors", "(joystick) Joystick control", "_Timer", "Setup manipulator", "(auto) Count balls", "(auto) Analyze balls", "(auto) Dot Controller", "Wait for button"] ("task")
              }
              frame "(mod) pattern" {
                w469 = T33 [enum."Setup get", enum."_Timer", enum."(image) get", enum."(pattern) Find Square", enum."(pattern) Calculate ROI", enum."(pattern) Analyze pattern", enum."Compare", enum."(pattern) Calc pattern indx", enum."(image) show", enum."(myRIO) update ports", enum."Wait for button"] items=["(qsm) schedule", "(qsm) initialize", "(qsm) release", "(qsm) clean up", "(qsm) shutdown", "(myRIO) initialize", "(myRIO) clean up", "(myRIO) update ports", "Setup get", "(image) get", "(image) show", "(ball) Shape detection", "(ball) Calc ball indx", "(ball) Calculate ROI", "(ball) Analyze color", "(ball) Align", "(ball) Wait", "(ball) Grab", "(pattern) Find Square", "(pattern) Calculate ROI", "(pattern) Calc pattern indx", "Compare", "(pattern) Analyze pattern", "(pattern) Align", "(pattern) Wait", "(pattern) states control", "navx", "stop motors", "(joystick) Joystick control", "_Timer", "Setup manipulator", "(auto) Count balls", "(auto) Analyze balls", "(auto) Dot Controller", "Wait for button"] ("task")
              }
              frame "<mod>[P] remembering" {
                w470 = T33 [enum."Setup get", enum."_Timer", enum."(image) get", enum."(pattern) Find Square", enum."(pattern) Calculate ROI", enum."(pattern) Analyze pattern", enum."(pattern) Calc pattern indx", enum."(image) show", enum."(myRIO) update ports", enum."Wait for button", enum."(pattern) states control"] items=["(qsm) schedule", "(qsm) initialize", "(qsm) release", "(qsm) clean up", "(qsm) shutdown", "(myRIO) initialize", "(myRIO) clean up", "(myRIO) update ports", "Setup get", "(image) get", "(image) show", "(ball) Shape detection", "(ball) Calc ball indx", "(ball) Calculate ROI", "(ball) Analyze color", "(ball) Align", "(ball) Wait", "(ball) Grab", "(pattern) Find Square", "(pattern) Calculate ROI", "(pattern) Calc pattern indx", "Compare", "(pattern) Analyze pattern", "(pattern) Align", "(pattern) Wait", "(pattern) states control", "navx", "stop motors", "(joystick) Joystick control", "_Timer", "Setup manipulator", "(auto) Count balls", "(auto) Analyze balls", "(auto) Dot Controller", "Wait for button"] ("task")
              }
              frame "<mod>[P] go through tunnel" {
                w471 = T33 [enum."Setup get", enum."_Timer", enum."(image) get", enum."(pattern) Find Square", enum."(pattern) Calculate ROI", enum."(pattern) Analyze pattern", enum."(pattern) Calc pattern indx", enum."(image) show", enum."(myRIO) update ports", enum."Wait for button", enum."(pattern) states control"] items=["(qsm) schedule", "(qsm) initialize", "(qsm) release", "(qsm) clean up", "(qsm) shutdown", "(myRIO) initialize", "(myRIO) clean up", "(myRIO) update ports", "Setup get", "(image) get", "(image) show", "(ball) Shape detection", "(ball) Calc ball indx", "(ball) Calculate ROI", "(ball) Analyze color", "(ball) Align", "(ball) Wait", "(ball) Grab", "(pattern) Find Square", "(pattern) Calculate ROI", "(pattern) Calc pattern indx", "Compare", "(pattern) Analyze pattern", "(pattern) Align", "(pattern) Wait", "(pattern) states control", "navx", "stop motors", "(joystick) Joystick control", "_Timer", "Setup manipulator", "(auto) Count balls", "(auto) Analyze balls", "(auto) Dot Controller", "Wait for button"] ("task")
              }
              frame "<mod>[P] comparing" {
                w472 = T33 [enum."Setup get", enum."_Timer", enum."(image) get", enum."(pattern) Find Square", enum."(qsm) schedule", enum."(pattern) Calculate ROI", enum."(pattern) Analyze pattern", enum."(pattern) Calc pattern indx", enum."(image) show", enum."(myRIO) update ports", enum."Wait for button", enum."(pattern) states control"] items=["(qsm) schedule", "(qsm) initialize", "(qsm) release", "(qsm) clean up", "(qsm) shutdown", "(myRIO) initialize", "(myRIO) clean up", "(myRIO) update ports", "Setup get", "(image) get", "(image) show", "(ball) Shape detection", "(ball) Calc ball indx", "(ball) Calculate ROI", "(ball) Analyze color", "(ball) Align", "(ball) Wait", "(ball) Grab", "(pattern) Find Square", "(pattern) Calculate ROI", "(pattern) Calc pattern indx", "Compare", "(pattern) Analyze pattern", "(pattern) Align", "(pattern) Wait", "(pattern) states control", "navx", "stop motors", "(joystick) Joystick control", "_Timer", "Setup manipulator", "(auto) Count balls", "(auto) Analyze balls", "(auto) Dot Controller", "Wait for button"] ("task")
              }
              frame "(mod) ball" {
                w473 = T33 [enum."(image) get", enum."(image) get", enum."(ball) Shape detection", enum."(ball) Calculate ROI", enum."(ball) Analyze color", enum."Compare", enum."(ball) Calc ball indx", enum."(image) show", enum."(myRIO) update ports", enum."Wait for button"] items=["(qsm) schedule", "(qsm) initialize", "(qsm) release", "(qsm) clean up", "(qsm) shutdown", "(myRIO) initialize", "(myRIO) clean up", "(myRIO) update ports", "Setup get", "(image) get", "(image) show", "(ball) Shape detection", "(ball) Calc ball indx", "(ball) Calculate ROI", "(ball) Analyze color", "(ball) Align", "(ball) Wait", "(ball) Grab", "(pattern) Find Square", "(pattern) Calculate ROI", "(pattern) Calc pattern indx", "Compare", "(pattern) Analyze pattern", "(pattern) Align", "(pattern) Wait", "(pattern) states control", "navx", "stop motors", "(joystick) Joystick control", "_Timer", "Setup manipulator", "(auto) Count balls", "(auto) Analyze balls", "(auto) Dot Controller", "Wait for button"] ("task")
              }
              frame "Ball" {
                w474 = T33 [enum."(image) get", enum."(ball) Shape detection", enum."(ball) Calculate ROI", enum."(ball) Calc ball indx", enum."(ball) Analyze color", enum."(image) show", enum."Wait for button", enum."(myRIO) update ports"] items=["(qsm) schedule", "(qsm) initialize", "(qsm) release", "(qsm) clean up", "(qsm) shutdown", "(myRIO) initialize", "(myRIO) clean up", "(myRIO) update ports", "Setup get", "(image) get", "(image) show", "(ball) Shape detection", "(ball) Calc ball indx", "(ball) Calculate ROI", "(ball) Analyze color", "(ball) Align", "(ball) Wait", "(ball) Grab", "(pattern) Find Square", "(pattern) Calculate ROI", "(pattern) Calc pattern indx", "Compare", "(pattern) Analyze pattern", "(pattern) Align", "(pattern) Wait", "(pattern) states control", "navx", "stop motors", "(joystick) Joystick control", "_Timer", "Setup manipulator", "(auto) Count balls", "(auto) Analyze balls", "(auto) Dot Controller", "Wait for button"] ("task")
              }
              frame "Other" {
                w475 = T33 [enum."(image) get", enum."(pattern) Find Square", enum."(pattern) Calculate ROI", enum."(pattern) Analyze pattern", enum."(image) show", enum."Wait for button", enum."(myRIO) update ports", enum."(image) get", enum."(ball) Shape detection", enum."(ball) Calculate ROI", enum."(ball) Analyze color", enum."(image) show", enum."Wait for button", enum."(myRIO) update ports"] items=["(qsm) schedule", "(qsm) initialize", "(qsm) release", "(qsm) clean up", "(qsm) shutdown", "(myRIO) initialize", "(myRIO) clean up", "(myRIO) update ports", "Setup get", "(image) get", "(image) show", "(ball) Shape detection", "(ball) Calc ball indx", "(ball) Calculate ROI", "(ball) Analyze color", "(ball) Align", "(ball) Wait", "(ball) Grab", "(pattern) Find Square", "(pattern) Calculate ROI", "(pattern) Calc pattern indx", "Compare", "(pattern) Analyze pattern", "(pattern) Align", "(pattern) Wait", "(pattern) states control", "navx", "stop motors", "(joystick) Joystick control", "_Timer", "Setup manipulator", "(auto) Count balls", "(auto) Analyze balls", "(auto) Dot Controller", "Wait for button"] ("task")
              }
              frame "Clear" {
                w476 = T33 [enum."Setup get", enum."(image) get", enum."(ball) Shape detection", enum."(ball) Calculate ROI", enum."(ball) Calc ball indx", enum."(ball) Analyze color", enum."(image) show", enum."(ball) Grab", enum."Wait for button", enum."(myRIO) update ports"] items=["(qsm) schedule", "(qsm) initialize", "(qsm) release", "(qsm) clean up", "(qsm) shutdown", "(myRIO) initialize", "(myRIO) clean up", "(myRIO) update ports", "Setup get", "(image) get", "(image) show", "(ball) Shape detection", "(ball) Calc ball indx", "(ball) Calculate ROI", "(ball) Analyze color", "(ball) Align", "(ball) Wait", "(ball) Grab", "(pattern) Find Square", "(pattern) Calculate ROI", "(pattern) Calc pattern indx", "Compare", "(pattern) Analyze pattern", "(pattern) Align", "(pattern) Wait", "(pattern) states control", "navx", "stop motors", "(joystick) Joystick control", "_Timer", "Setup manipulator", "(auto) Count balls", "(auto) Analyze balls", "(auto) Dot Controller", "Wait for button"] ("task")
              }
              frame "(auto) Balls Analyze" {
                w477 = T33 [enum."(image) get", enum."(ball) Shape detection", enum."(auto) Count balls", enum."(auto) Analyze balls", enum."Wait for button", enum."(myRIO) update ports"] items=["(qsm) schedule", "(qsm) initialize", "(qsm) release", "(qsm) clean up", "(qsm) shutdown", "(myRIO) initialize", "(myRIO) clean up", "(myRIO) update ports", "Setup get", "(image) get", "(image) show", "(ball) Shape detection", "(ball) Calc ball indx", "(ball) Calculate ROI", "(ball) Analyze color", "(ball) Align", "(ball) Wait", "(ball) Grab", "(pattern) Find Square", "(pattern) Calculate ROI", "(pattern) Calc pattern indx", "Compare", "(pattern) Analyze pattern", "(pattern) Align", "(pattern) Wait", "(pattern) states control", "navx", "stop motors", "(joystick) Joystick control", "_Timer", "Setup manipulator", "(auto) Count balls", "(auto) Analyze balls", "(auto) Dot Controller", "Wait for button"] ("task")
              }
              frame "Joystick control" {
                w478 = T33 [enum."(joystick) Joystick control", enum."(myRIO) update ports"] items=["(qsm) schedule", "(qsm) initialize", "(qsm) release", "(qsm) clean up", "(qsm) shutdown", "(myRIO) initialize", "(myRIO) clean up", "(myRIO) update ports", "Setup get", "(image) get", "(image) show", "(ball) Shape detection", "(ball) Calc ball indx", "(ball) Calculate ROI", "(ball) Analyze color", "(ball) Align", "(ball) Wait", "(ball) Grab", "(pattern) Find Square", "(pattern) Calculate ROI", "(pattern) Calc pattern indx", "Compare", "(pattern) Analyze pattern", "(pattern) Align", "(pattern) Wait", "(pattern) states control", "navx", "stop motors", "(joystick) Joystick control", "_Timer", "Setup manipulator", "(auto) Count balls", "(auto) Analyze balls", "(auto) Dot Controller", "Wait for button"]
              }
              frame "navx" {
                w479 = T33 [enum."navx", enum."(myRIO) update ports"] items=["(qsm) schedule", "(qsm) initialize", "(qsm) release", "(qsm) clean up", "(qsm) shutdown", "(myRIO) initialize", "(myRIO) clean up", "(myRIO) update ports", "Setup get", "(image) get", "(image) show", "(ball) Shape detection", "(ball) Calc ball indx", "(ball) Calculate ROI", "(ball) Analyze color", "(ball) Align", "(ball) Wait", "(ball) Grab", "(pattern) Find Square", "(pattern) Calculate ROI", "(pattern) Calc pattern indx", "Compare", "(pattern) Analyze pattern", "(pattern) Align", "(pattern) Wait", "(pattern) states control", "navx", "stop motors", "(joystick) Joystick control", "_Timer", "Setup manipulator", "(auto) Count balls", "(auto) Analyze balls", "(auto) Dot Controller", "Wait for button"]
              }
            }
            n43 = call "enqueue_states.vi"("task"=w458, "error in"=w461, "queue in"=w462) -> ("error out"=w463:errorcluster)  [unwired: 6 in, 1 out]
          }
          frame "(qsm) initialize" {
            w493 = 30
            w496 = 20
            w505 = T34 0 items=["Grayscale (U8)", "Grayscale (I16)", "Grayscale (SGL)", "Complex (CSG)", "RGB (U32)", "HSL (U32)", "RGB (U64)", "Grayscale (U16)"] ("Image Type")
            # "Initialize -- Allocate memory for additional image buffers, if necessary, and perform other one-time initialization steps."
            n44 = Initialize Array(0 ("element"), "Dots in total") -> (→"Angles" →"Left_enc" →"Right_enc" →"M_enc" →"G_enc":i32[])
            n45 = local read "Dots in total"() -> (w486:i32)
            n46 = local read "States in total"() -> (w482:i32)
            n47 = Initialize Array(0 ("element"), "States in total", w486) -> (→"Dots of States":i32[][])
            n48 = Initialize Array(0 ("element"), w482) -> (→"FT_Angles" →"FT_Left_enc" →"FT_Right_enc" →"FT_M_enc" →"FT_G_enc":i32[])
            n49 = Unbundle By Name(w499) -> ("Color classes"=w497:i32[], "Pattern classes"=w492:i32[])
            n50 = call "IMAQ Create"("Border Size"=3, "Image Name"="img0", "Image Type"=w505, "error in (no error)"=w508) -> ("New Image"=w503:T7, "error out"=w507:errorcluster)  [unwired: 1 in]
            n51 = Insert Into Array(array=w497, index=0, new element #1=w496, new element #2=w496, new element #3=w496, new element #4=w496, new element #5=w496) -> (w495:i32[])
            n52 = Insert Into Array(array=w492, index=0, new element #1=w493, new element #2=w493, new element #3=w493, new element #4=w493, new element #5=w493) -> (w491:i32[])
            n53 = Bundle By Name(cluster=w499, "image ref"=w503) -> (w501:T10)
            n54 = Bundle By Name(cluster=w501, "Color classes"=w495, "Pattern classes"=w491) -> (w500:T10)
          }
          frame "(qsm) release" {
            # "Release all front-panel action buttons."
          }
          frame "(qsm) clean up" {
            # "Set the \"Stop webcam\" flag"
            # "Clean up -- Set the \"Stop webcam flag\" and perform other necessary clean-up actions."
            n55 = Bundle By Name(cluster=w517, "qsm.Stop webcam"=TRUE) -> (w516:T10)
          }
          frame "(qsm) shutdown" {
            # "deallocate image buffer memory"
            # "stop the loop"
            # "Shutdown -- Release the state queue, free all image buffer memory, and stop the while-loop structure."
            n56 = Release Queue(queue=w526, error in (no error)=w527) -> (error out=w523:errorcluster)  [unwired: 1 in, 2 out]
            n57 = call "Imaq Dispose"("All Images? (No)"=TRUE, "error in (no error)"=w523) -> ("error out"=w522:errorcluster)  [unwired: 4 in]
          }
          frame "(myRIO) initialize" {
            # "Initialize (myRIO) -- Open channels, configure devices, send setup strings to peripherals, etc."
          }
          frame "(myRIO) clean up" {
            w536 = FALSE ("LED3")
            # "clear the onboard LEDs"
            # "Clean up (myRIO) -- Return myRIO devices and external peripherals to inactive states."
            n58 = xnode "LED 3"("LED0"=w536, "LED1"=w536, "LED2"=w536, "LED3"=w536, "error in (no error)"=w535) -> ("error out"=w534:errorcluster)
          }
          frame "(myRIO) update ports" {
            # "show the button state\non the onboard LEDs"
            # "set the flag"
            # "press the onboard button\nto set the \"save image\" flag"
            # "Update ports (myRIO) -- Read and write onboard devices and external peripherals."
            n59 = xnode "Button"("error in (no error)"=w581) -> ("Value"=w578:bool, "error out"=w580:errorcluster)
            n60 = xnode "LED"("LED0"=w578, "LED1"=w578, "LED2"=w578, "LED3"=w578, "error in (no error)"=w580) -> ("error out"=w579:errorcluster)
          }
          frame "Setup get" {
            n61 = Unbundle By Name(w668) -> ("Shape - t, Color - f"=w662:T30)
            n62 = case shown="\"Pattern\"" w662 {
              frame "Align", Default {
                n63 = local write "Camera state"(enum16{"Fwd", "Pattern", "Ball"}."Ball" ("Camera state")) -> ()
                "rotate" <- FALSE ("rotate")
              }
              frame "(pattern) Align" {
                n64 = local write "rotate"(TRUE ("rotate")) -> ()
                n65 = local write "Camera state"(enum16{"Fwd", "Pattern", "Ball"}."Pattern" ("Camera state")) -> ()
              }
              frame "Pattern" {
                n66 = local write "Camera state"(enum16{"Fwd", "Pattern", "Ball"}."Pattern" ("Camera state")) -> ()
              }
              frame "(mod) pattern" {
                n67 = local write "Camera state"(enum16{"Fwd", "Pattern", "Ball"}."Pattern" ("Camera state")) -> ()
              }
              frame "<mod>[P] remembering" {
                n68 = local write "Camera state"(enum16{"Fwd", "Pattern", "Ball"}."Pattern" ("Camera state")) -> ()
              }
              frame "<mod>[P] go through tunnel" {
                n69 = local write "Camera state"(enum16{"Fwd", "Pattern", "Ball"}."Pattern" ("Camera state")) -> ()
              }
              frame "<mod>[P] comparing" {
                n70 = local write "Camera state"(enum16{"Fwd", "Pattern", "Ball"}."Pattern" ("Camera state")) -> ()
              }
              frame "(mod) ball" {
                n71 = local write "Camera state"(enum16{"Fwd", "Pattern", "Ball"}."Ball" ("Camera state")) -> ()
              }
              frame "Ball" {
                n72 = local write "Camera state"(enum16{"Fwd", "Pattern", "Ball"}."Ball" ("Camera state")) -> ()
              }
              frame "Other" {
              }
              frame "Clear" {
                n73 = local write "Camera state"(enum16{"Fwd", "Pattern", "Ball"}."Ball" ("Camera state")) -> ()
              }
              frame "navx" {
              }
              frame "Joystick control" {
              }
            }
            n74 = call "Setup camera (SubVI).vi"("M duty cycle [P]"="M duty cycle [P]", "S duty cycle [B]   in"="S duty cycle [B]", "M duty cycle [B]  in"="M duty cycle [B]", "S duty cycle [F]"="S duty cycle [F]", "M duty cycle [F]"="M duty cycle [F]", "Camera state"="Camera state", "S duty cycle [P]"="S duty cycle [P]") -> ("M duty cycle [B]  out"=w664:dbl, "S duty cycle [B]   out"=w663:dbl)  [unwired: 3 in]
            n75 = local write "[cur] duty cycle [%] (s)"(w663) -> ()
            n76 = local write "[cur] duty cycle [%] (m)"(w664) -> ()
          }
          frame "(image) get" {
            # "NOTE:\n1. Use NI-MAX to configure your webcam with the\n     *same* resolution (\"mode\") and attributes as those used \n     to develop your Vision Assistant script, especially if the\n     script depends on absolute ROIs, calibration images, template\n     images, background levels, etc.\n \n     Click \"Save\" to create or update the camera configuration files\n     on the target.\n\n2. Open the Vision Acquisition Express VI above and then\n     select \"Reset to Defaults\" to read the camera configuration\n     files created/updated by NI-MAX in the previous step."
            # "webcam image buffer is\ncreated during the first\ncall of the Vision\nAcquisition Express VI"
            # "Get image -- Retrieve a single webcam image frame and optionally flip the image right side up."
            n77 = call "Vision Acquisition"("error in"=w691) -> ("Image Out"=w689:T7, "error out"=w690:errorcluster)  [unwired: 24 in, 1 out]
            n78 = local read "rotate"() -> (w692:bool)
            n79 = case shown="False" w692 {
              tunnel: w689 -> [w703 w708]
              tunnel: [w703 w707] -> w687
              tunnel: w690 -> [w702 w705]
              tunnel: [w702 w706] -> w686
              frame False {
                # "use webcam image as-is"
              }
              frame True {
                # "rotate img for pattern"
                n80 = call "IMAQ Rotate"("error in (no error)"=w705, "Angle (degrees)"="Angle for pattern (degrees)", "Image Src"=w708) -> ("error out"=w706:errorcluster, "Image Dst Out"=w707:T7)  [unwired: 7 in]
              }
            }
            n81 = Unbundle By Name(w683) -> ("Shape - t, Color - f"=w682:T30)
            n82 = case shown="\"Align\", Default" w682 {
              tunnel: w687 -> [w696 w701]
              tunnel: w686 -> [w695 w698]
              tunnel: [w696 w700] -> w685
              tunnel: [w695 w699] -> w684
              frame "Align", Default {
              }
              frame "(pattern) Align" {
                n83 = call "IMAQ Rotate"("error in (no error)"=w698, "Angle (degrees)"="Angle for Align (degrees)", "Image Src"=w701) -> ("error out"=w699:errorcluster, "Image Dst Out"=w700:T7)  [unwired: 7 in]
              }
            }
            n84 = Bundle By Name(cluster=w693, "qsm.Webcam image ref"=w685) -> (w694:T10)
          }
          frame "(image) show" {
            # "Show image -- Select from among the available image buffers to show on the main image display; use a selector tree or case structure."
            n85 = Unbundle By Name "Unbundle By Name"(w712) -> ("show analyzed"=w711:bool)
            n86 = Unbundle By Name "Unbundle By Name"(w714) -> ("qsm.Analyzed image ref"=w717:T7, "qsm.Webcam image ref"=w716:T7)
            n87 = Select(t=w717, s=w711, f=w716) -> (s? t:f=→"image display":T7)
          }
          frame "(ball) Shape detection" {
            # "Shape detection"
            # "Expansion State A"
            n88 = Unbundle By Name(w732) -> ("qsm.Webcam image ref"=w734:T7)
            n89 = call "Vision Assistant"("Image In"=w734, "error in"=w735) -> ("Image Out"=w733:T7, "error out"=w730:errorcluster, "Circles Calibrated (Shape Detection 1)"=w728:T3, "Number of Matches (Shape Detection 1)"=→"Number of Matches (Shape Detection 1)":i32)  [unwired: 22 in]
            "Circles Calibrated (Shape Detection 1)" <- w728
            n90 = Index Array(array=w728, index=0) -> (element=w725:T35)
            n91 = Unbundle By Name(w725) -> ("Position"=w724:cluster{"X":sgl, "Y":sgl}, "Radius"=→"CircleRadius":dbl)
            n92 = Unbundle(w724) -> ("X"=w723:sgl, "Y"=w722:sgl)
            n93 = To Double Precision Float(number=w723) -> (double precision float=→"curX":dbl)
            n94 = To Double Precision Float(number=w722) -> (double precision float=→"curY":dbl)
            n95 = Bundle By Name(cluster=w732, "qsm.Analyzed image ref"=w733) -> (w731:T10)
          }
          frame "(ball) Calc ball indx" {
            n96 = Unbundle By Name(w740) -> ("Shape - t, Color - f"=w737:T30)
            n97 = Equal?(x=w737, y=T29."(mod) ball" ("Shape - t, Color - f")) -> (x = y?=w739:bool)
            n98 = case shown="False" w739 {
              frame False {
                n99 = local read "Circles Calibrated (Shape Detection 1)"() -> (w747:T3)
                n100 = control-ref of="Ball number"() -> (w749:refnum<vi>)
                n101 = control-ref of="Number of Matches (Shape Detection 1)"() -> (w750:refnum<vi>)
                n102 = local read "curX"() -> (w746:dbl)
                n103 = local read "curY"() -> (w745:dbl)
                n104 = To Single Precision Float(number=w746) -> (single precision float=w744:sgl)
                n105 = To Single Precision Float(number=w745) -> (single precision float=w743:sgl)
                n106 = call "Ball Index (SubVI).vi"("cur pos Y"=w743, "cur pos X"=w744, "Circles Calibrated (Shape Detection 1)"=w747, "Ball index"="Ball number", "reference in"=w749, "Digital in"=w750) -> ()  [unwired: 4 in]
              }
              frame True {
                n107 = local read "Ball number"() -> (w752:i32)
                n108 = Increment(x=w752) -> (x+1=w751:i32)
                n109 = local write "Ball number"(w751) -> ()
              }
            }
          }
          frame "(ball) Calculate ROI" {
            n110 = local read "Number of Matches (Shape Detection 1)"() -> (w764:i32)
            n111 = Greater Than 0?(x=w764) -> (x > 0?=w761:bool)
            n112 = local read "curX"() -> (w763:dbl)
            n113 = local read "curY"() -> (w762:dbl)
            n114 = local read "ROI Descriptor COLOR"() -> (w755:T4)
            n115 = local read "CircleRadius"() -> (w753:dbl)
            n116 = call "Ball ROI (SubVI).vi"("ROI Descriptor COLOR Mask"=w755, "divider (circle)"="divider (circle)", "curY"=w762, "curX"=w763, "Boolean"=w761, "Radius"=w753) -> ("x1"=→"x1 (circle)":i32, "y0"=→"y0 (circle)":i32, "x0"=→"x0 (circle)":i32, "ROI Descriptor COLOR Mask out"=w756:T4, "y1"=→"y1 (circle)":i32)  [unwired: 1 in]
            n117 = local write "ROI Descriptor COLOR"(w756) -> ()
          }
          frame "(ball) Analyze color" {
            # "Color analyze"
            # "analyzed image buffer is\ncreated during the first\ncall of the Vision\nAssistant Express VI *only*\nwhen \"Create Destination\nImage\" option is enabled"
            # "Analyze image -- Analyze the webcam image with a Vision Assistant script."
            n118 = Unbundle By Name "Unbundle By Name"(w784) -> ("Color classes"=w778:i32[], "qsm.Webcam image ref"=w775:T7)
            n119 = call "Vision Assistant2"("Image In"=w775, "error in"=w772, "ROI Descriptor (Image Mask 1)"="ROI Descriptor COLOR", "ROI Descriptor (Color Classification 1)"="ROI Descriptor COLOR") -> ("Image Out"=w773:T7, "error out"=w771:errorcluster, "Classes (Color Classification 1)"=w774:string[])  [unwired: 21 in]
            n120 = Index Array(array=w774, index=0) -> (element=w782:string)
            n121 = local read "Ball number"() -> (w776:i32)
            n122 = Decimal String To Number(string=w782) -> (number=w777:i32)  [unwired: 2 in, 1 out]
            "Color" <- w777
            n123 = Insert Into Array(array=w778, index=w776, new element=w777) -> (w779:i32[])
            n124 = Bundle By Name "Bundle By Name"(cluster=w784, "qsm.Analyzed image ref"=w773, "Color class"=w777, "Color classes"=w779) -> (w783:T10)
          }
          frame "(ball) Align" {
            # "Align"
            # "Expansion State B"
            n125 = flat-sequence {
              frame #0 {
                w789 = FALSE ("X is in range")
                n126 = local write "X is in range"(w789) -> ()
                n127 = local write "Y is in range"(w789) -> ()
              }
              frame #1 {
                n128 = local read "Y is in range"() -> (w795:bool)
                n129 = local read "X is in range"() -> (w796:bool)
                n130 = local read "L_PWM"() -> (w791:dbl)
                n131 = local read "R_PWM"() -> (w790:dbl)
                n132 = local read "curX"() -> (w806:dbl)
                n133 = local read "curY"() -> (w803:dbl)
                n134 = call "Ball Align(SubVI).vi"("Align X - t, Y - f"="Align X - t, Y - f", "x is in range"=w796, "y is in range"=w795, "L_PWM"=w791, "R_PWM"=w790, "curX"=w806, "defY"="defY", "curY"=w803, "defX"="defX", "Range"="Range") -> ("x_is_in_range"=→"X is in range":bool, "y_is_in_range"=→"Y is in range":bool, "Align_X-t,Y-f"=w794:bool, "Boolean 4"=w800:bool, "Boolean"=w797:bool, "Boolean 3"=w799:bool, "Boolean 2"=w798:bool, "L_PWM out"=w793:dbl, "R_PWM out"=w792:dbl)  [unwired: 9 in]
                n135 = local write "Align X - t, Y - f"(w794) -> ()
                n136 = local write "R_PWM"(w792) -> ()
                n137 = local write "L_PWM"(w793) -> ()
                n138 = local write "Right+"(w799) -> ()
                n139 = local write "Right-"(w798) -> ()
                n140 = local write "Left-"(w800) -> ()
                n141 = local write "Left+"(w797) -> ()
              }
            }
          }
          frame "(ball) Wait" {
            # "Expansion State D"
            n142 = flat-sequence {
              frame #0 {
                n143 = Wait (ms)(milliseconds to wait="align accuracy") -> ()  [unwired: 1 out]
              }
              frame #1 {
                w821 = FALSE
                n144 = local write "Left-"(w821) -> ()
                n145 = local write "Left+"(w821) -> ()
                n146 = local write "Right+"(w821) -> ()
                n147 = local write "Right-"(w821) -> ()
              }
            }
            n148 = local read "X is in range"() -> (w818:bool)
            n149 = local read "Y is in range"() -> (w817:bool)
            n150 = And(x=w818, y=w817) -> (x .and. y?=w819:bool)
            n151 = case shown="False" w819 {
              tunnel: w816 -> [w826 w831]
              tunnel: [w826 w831] -> w815
              tunnel: w814 -> [w825 w829]
              tunnel: [w823 w828] -> w813
              tunnel: w812 -> [w824 w830]
              tunnel: [w824 w830] -> w811
              tunnel: w810 -> [_ _]
              frame False {
                n152 = Bundle By Name(cluster=w825, "Shape - t, Color - f"=T30."Align") -> (w823:T8)
              }
              frame True {
                n153 = Bundle By Name(cluster=w829, "Shape - t, Color - f"=T30."Clear") -> (w828:T8)
              }
            }
          }
          frame "(ball) Grab" {
            # "Expansion State E"
            n154 = call "Setup manipulator (SubVI).vi"("Release?"=FALSE, "G_upper bound"="G_UB_grab", "M_lower bound"="M_UB_grab", "error in (no error)"=w841, "M_Encoder Ref In"=w839, "G_Encoder Ref In"=w838) -> ("error out"=w840:errorcluster)  [unwired: 9 in]
            n155 = Bundle By Name(cluster=w834, "Shape - t, Color - f"=T30."Align") -> (w833:T8)
          }
          frame "(pattern) Find Square" {
            # "analyzed image buffer is\ncreated during the first\ncall of the Vision\nAssistant Express VI *only*\nwhen \"Create Destination\nImage\" option is enabled"
            # "Expansion State F"
            n156 = Unbundle By Name "Unbundle By Name"(w844) -> ("qsm.Webcam image ref"=w862:T7)
            n157 = call "Vision Assistant3"("Image In"=w862, "error in"=w859) -> ("Image Out"=w857:T7, "error out"=w860:errorcluster, "Calibrated Matches (Geometric Matching 1)"=w856:T5[], "Number of Matches (Geometric Matching 1)"=→"Number of Matches (Geometric Matching 1)":i32)  [unwired: 22 in]
            "Calibrated Matches (Geometric Matching 1)" <- w856
            n158 = Bundle By Name(cluster=w844, "qsm.Analyzed image ref"=w857) -> (w858:T10)
            n159 = Index Array(array=w856, index=0) -> (element=w854:T5)
            n160 = Unbundle By Name(w854) -> ("Position"=w853:cluster{"x":sgl, "y":sgl})
            n161 = Unbundle By Name(w853) -> ("x"=→"curX(p)":sgl)
            n162 = Unbundle By Name(w848) -> ("Shape - t, Color - f"=w847:T30)
            n163 = Equal?(x=w847, y=T31."<mod>[P] comparing") -> (x = y?=w851:bool)
            n164 = case shown="True" w851 {
              tunnel: [w863 T31."(pattern) Align" ("Shape - t, Color - f")] -> w849
              tunnel: w847 -> [w863 _]
              frame False {
              }
              frame True {
              }
            }
            n165 = Bundle By Name(cluster=w848, "Shape - t, Color - f"=w849) -> (w850:T8)
          }
          frame "(pattern) Calculate ROI" {
            # "Expansion State G"
            n166 = local read "Number of Matches (Geometric Matching 1)"() -> (w876:i32)
            n167 = local read "Calibrated Matches (Geometric Matching 1)"() -> (w875:T5[])
            n168 = Unbundle By Name(w878) -> ("ROI Descriptor (Image Mask 1).Contours"=w868:T36)
            n169 = Greater Than 0?(x=w876) -> (x > 0?=w880:bool)
            n170 = call "Pattern ROI (SubVI).vi"("y"="divider (pattern)", "Boolean"=w880, "Calibrated Matches (Geometric Matching 1)"=w875, "Contours in"=w868) -> ("Numeric 4"=→"y1":i32, "Numeric 3"=→"x1":i32, "Numeric"=→"y0":i32, "Scale"=→"Scale":sgl, "Numeric 2"=→"x0":i32, "Contours out"=w867:T36)  [unwired: 2 in]
            n171 = Bundle By Name(cluster=w878, "ROI Descriptor (Image Mask 1).Contours"=w867) -> (w866:T10)
          }
          frame "(pattern) Calc pattern indx" {
            n172 = local read "pattern number"() -> (w883:i32)
            n173 = Increment(x=w883) -> (x+1=w882:i32)
            n174 = local write "pattern number"(w882) -> ()
          }
          frame "Compare" {
            n175 = Unbundle By Name(w892) -> ("Shape - t, Color - f"=w891:T30)
            n176 = Equal?(x=w891, y=T32."(mod) ball") -> (x = y?=w889:bool)
            n177 = Not(x=w889) -> (.not. x?=w888:bool)
            n178 = case shown="False" w888 {
              tunnel: w893 -> [w898 w904]
              frame False {
                n179 = local read "Ball number"() -> (w899:i32)
                n180 = control-ref of="ball match"() -> (w896:refnum<vi>)
                n181 = Unbundle By Name(w898) -> ("Color classes"=w897:i32[])
                n182 = Greater?(x=w899, y="Balls to remember") -> (0:w901:bool)
                n183 = call "(ball) Compare (SubVI).vi"("Boolean"=w901, "Balls to remember"="Balls to remember", "Ball number"=w899, "Color classes"=w897, "Boolean in"=w896) -> ("ball match"=→"ball match":bool)  [unwired: 6 in]
              }
              frame True {
                n184 = local read "pattern number"() -> (w902:i32)
                n185 = Greater?(x=w902, y="patterns to remember") -> (0:w906:bool)
                n186 = Unbundle By Name(w904) -> ("Pattern classes"=w903:i32[])
                n187 = case shown="True" w906 {
                  tunnel: "patterns to remember" -> [_ w910]
                  tunnel: w903 -> [_ w908]
                  tunnel: w902 -> [_ w907]
                  frame False {
                  }
                  frame True {
                    n188 = flat-sequence {
                      tunnel: w910 -> [w912]
                      tunnel: [w912] -> w909
                      tunnel: w909 -> [w915]
                      tunnel: w908 -> [w914]
                      tunnel: w907 -> [w913]
                      frame #0 {
                        n189 = local write "pattern match"(FALSE ("pattern match")) -> ()
                      }
                      frame #1 {
                        n190 = for {
                          N: w915 -> [_]
                          tunnel: w913 -> [w924]
                          tunnel: w914 -> [w918]
                          i -> [w920]
                          n191 = Increment(x=w920) -> (x+1=w919:i32)
                          n192 = Index Array(array=w918, index=w919) -> (element=w917:i32)
                          n193 = Index Array(array=w918, index=w924) -> (element=w916:i32)
                          n194 = Equal?(x=w917, y=w916) -> (x = y?=w923:bool)
                          n195 = local read "pattern match"() -> (w922:bool)
                          n196 = Not(x=w922) -> (.not. x?=w921:bool)
                          n197 = case shown="True" w921 {
                            tunnel: w923 -> [_ w925]
                            frame False {
                            }
                            frame True {
                              "pattern match" <- w925
                            }
                          }
                        }
                      }
                    }
                  }
                }
              }
            }
          }
          frame "(pattern) Analyze pattern" {
            n198 = Unbundle By Name(w935) -> ("Pattern classes"=w929:i32[], "qsm.Webcam image ref"=w939:T7, "ROI Descriptor (Image Mask 1)"=w933:T4)
            n199 = call "Vision Assistant4"("Image In"=w939, "error in"=w937, "ROI Descriptor (Image Mask 1)"=w933, "ROI Descriptor (Particle Classification 1)"=w933) -> ("Image Out"=w938:T7, "error out"=w936:errorcluster, "Class (Particle Classification 1)"=w928:string)  [unwired: 21 in]
            n200 = Decimal String To Number(string=w928) -> (number=w927:i32)  [unwired: 2 in, 1 out]
            "Pattern" <- w927
            n201 = Insert Into Array(array=w929, index="pattern number", new element=w927) -> (w931:i32[])
            n202 = Bundle By Name(cluster=w935, "qsm.Analyzed image ref"=w938, "Pattern classes"=w931) -> (w934:T10)
          }
          frame "(pattern) Align" {
            # "Bck"
            # "Fwd"
            n203 = local read "curX(p)"() -> (w943:sgl)
            n204 = call "Pattern Align(SubVI).vi"("curX(p)"=w943, "defX(p)"="defX(p)", "Range(p)"="Range(p)") -> ("In Range?"=→"In Range? (p)":bool, "Bck"=w946:bool, "Fwd"=w945:bool)  [unwired: 6 in]
            n205 = local write "Right+"(w945) -> ()
            n206 = local write "Right-"(w946) -> ()
            n207 = local write "Left+"(w945) -> ()
            n208 = local write "Left-"(w946) -> ()
          }
          frame "(pattern) Wait" {
            n209 = flat-sequence {
              tunnel: [w959] -> w952
              tunnel: w951 -> [w958]
              frame #0 {
                n210 = Wait (ms)(milliseconds to wait="align accuracy (p)") -> ()  [unwired: 1 out]
              }
              frame #1 {
                w957 = FALSE ("Right+")
                n211 = local write "Right+"(w957) -> ()
                n212 = local write "Right-"(w957) -> ()
                n213 = local write "Left+"(w957) -> ()
                n214 = local write "Left-"(w957) -> ()
              }
              frame #2 {
                n215 = local read "In Range? (p)"() -> (w960:bool)
                n216 = Equal?(x=".Task", y=enum16{"Def", "<mod>[P]+tnl "}."<mod>[P]+tnl ") -> (x = y?=w962:bool)
                n217 = And(x=w960, y=w962) -> (x .and. y?=w961:bool)
                n218 = case shown="False" w961 {
                  tunnel: [T31."(pattern) Align" ("Shape - t, Color - f") w967] -> w959
                  tunnel: w958 -> [_ w966]
                  frame False {
                  }
                  frame True {
                    n219 = Unbundle By Name(w966) -> ("Shape - t, Color - f"=w967:T30)
                  }
                }
              }
            }
            n220 = Bundle By Name(cluster=w951, "Shape - t, Color - f"=w952) -> (w953:T8)
          }
          frame "(pattern) states control" {
            n221 = flat-sequence {
              tunnel: w970 -> [w977]
              tunnel: w970 -> [w976]
              tunnel: [w975] -> w969
              frame #0 {
                n222 = Increment(x=",ctl num") -> (x+1=w973:i32)
                n223 = local write ",ctl num"(w973) -> ()
              }
              frame #1 {
                n224 = Unbundle By Name(w977) -> ("Shape - t, Color - f"=w978:T30)
                n225 = case shown="\"(auto) Balls Analyze\"" w978 {
                  tunnel: w976 -> [w981 w990 w999 w1005 w1006 w1007 w1008 w1009 w1010 w1011 w1012 w1013 w1014 w1015]
                  tunnel: [w980 w989 w999 w1005 w1006 w1007 w1008 w1009 w1010 w1011 w1012 w1013 w1014 w1015] -> w975
                  frame "<mod>[P] remembering" {
                    n226 = local read ",ctl num"() -> (w983:i32)
                    n227 = Greater?(x=w983, y=3) -> (0:w979:bool)
                    n228 = case shown="True" w979 {
                      tunnel: w981 -> [w984 w988]
                      tunnel: [w984 w987] -> w980
                      frame False {
                      }
                      frame True {
                        n229 = Bundle By Name(cluster=w988, "Shape - t, Color - f"=T30."<mod>[P] go through tunnel") -> (w987:T8)
                        n230 = local write ",ctl num"(0 ("ctl num")) -> ()
                      }
                    }
                  }
                  frame "<mod>[P] go through tunnel" {
                    n231 = local read ",ctl num"() -> (w993:i32)
                    n232 = Greater?(x=w993, y=1) -> (0:w991:bool)
                    n233 = case shown="True" w991 {
                      tunnel: w990 -> [w994 w998]
                      tunnel: [w994 w997] -> w989
                      frame False {
                      }
                      frame True {
                        n234 = Bundle By Name(cluster=w998, "Shape - t, Color - f"=T30."<mod>[P] comparing") -> (w997:T8)
                        n235 = local write ",ctl num"(0 (",ctl num")) -> ()
                      }
                    }
                  }
                  frame "<mod>[P] comparing" {
                    n236 = local read ",ctl num"() -> (w1001:i32)
                    n237 = Greater?(x=w1001, y=5) -> (0:w1002:bool)
                    n238 = case shown="True" w1002 {
                      frame False {
                      }
                      frame True {
                        n239 = local write ",ctl num"(0 (",ctl num")) -> ()
                        n240 = local write "Stop"(TRUE ("Stop")) -> ()
                      }
                    }
                  }
                  frame "(mod) ball" {
                  }
                  frame "Ball" {
                  }
                  frame "Other" {
                  }
                  frame "Clear" {
                  }
                  frame "(auto) Balls Analyze" {
                  }
                  frame "Joystick control" {
                  }
                  frame "(mod) pattern" {
                  }
                  frame "Pattern" {
                  }
                  frame "(pattern) Align" {
                  }
                  frame "Align" {
                  }
                  frame "navx" {
                  }
                }
              }
            }
          }
          frame "navx" {
            n241 = disable-structure shown="Disabled" {
              disable-tunnel: w1018 -> [w1035 _]
              disable-tunnel: [w1034 _] -> w1017
              disable-tunnel: [w1031 _] -> w1016
              frame Disabled {
                n242 = call "sonic info (SubVI).vi"("error in (no error)"=w1035) -> ("error out"=w1034:errorcluster, "distance to the side"=w1033:u32)  [unwired: 9 in]
                "distance to the side" <- w1033
                n243 = Less Or Equal?(x=w1033, y=u32 7) -> (x <= y?=w1031:bool)
              }
              frame Enabled {
              }
            }
            n244 = disable-structure shown="Disabled" {
              disable-tunnel: _ -> [w1045 _]
              disable-tunnel: _ -> [w1044 _]
              disable-tunnel: [w1043 _] -> _
              disable-tunnel: [w1037 _] -> _
              disable-tunnel: [w1036 _] -> _
              frame Disabled {
                n245 = control-ref of="Left+"() -> (w1042:refnum<vi>)
                n246 = control-ref of="Left-"() -> (w1041:refnum<vi>)
                n247 = control-ref of="Right+"() -> (w1040:refnum<vi>)
                n248 = control-ref of="Right-"() -> (w1039:refnum<vi>)
                n249 = call "align.vi"("Right-"=w1039, "I2C Ref Out"=w1045, "error in (no error)"=w1044, "Right+"=w1040, "Left-"=w1041, "Left+"=w1042) -> ("error out"=w1037:errorcluster, "Aligned"=w1036:bool, "value Z"=→"value Z":ext, "I2C Ref Out out"=w1043:T22)  [unwired: 2 in]
              }
              frame Enabled {
              }
            }
            n250 = control-ref of="L_PWM"() -> (w1026:refnum<vi>)
            n251 = control-ref of="R_PWM"() -> (w1025:refnum<vi>)
            n252 = call "fwd-navx (SubVI).vi"("error in (no error)"=w1017, "I2C Ref Out"=w1023, "R_PWM"=w1025, "L_PWM"=w1026) -> ("error out"=w1027:errorcluster, "I2C Ref Out out"=w1028:T22, "value Z"=→"value Z 2":ext, "Right+"=w1022:bool, "Left+"=w1021:bool)  [unwired: 3 in]
            n253 = Not(x=w1021) -> (.not. x?=w1020:bool)
            n254 = Not(x=w1022) -> (.not. x?=w1019:bool)
            n255 = local write "Left+"(w1021) -> ()
            n256 = local write "Right+"(w1022) -> ()
            n257 = local write "Left-"(w1020) -> ()
            n258 = local write "Right-"(w1019) -> ()
          }
          frame "stop motors" {
            n259 = flat-sequence {
              frame #0 {
                w1050 = TRUE ("Right+")
                n260 = local write "Left+"(w1050) -> ()
                n261 = local write "Left-"(w1050) -> ()
                n262 = local write "Right+"(w1050) -> ()
                n263 = local write "Right-"(w1050) -> ()
              }
              frame #1 {
                w1051 = FALSE ("Right+")
                n264 = local write "Left+"(w1051) -> ()
                n265 = local write "Left-"(w1051) -> ()
                n266 = local write "Right+"(w1051) -> ()
                n267 = local write "Right-"(w1051) -> ()
              }
            }
          }
          frame "(joystick) Joystick control" {
            n268 = shared-variable "My Computer\\KeyLibrary.lvlib\\Power"() -> (w1053:dbl)  [unwired: 1 in, 1 out]
            n269 = call "Joystick control (SubVI).vi"() -> ("G+"=w1060:bool, "M-"=w1062:bool, "M+"=w1061:bool, "G-"=w1059:bool, "Left+"=w1055:bool, "Right-"=w1054:bool, "Left-"=w1056:bool, "Right+"=w1057:bool)  [unwired: 4 in]
            n270 = local write "L_PWM"(w1053) -> ()
            n271 = local write "R_PWM"(w1053) -> ()
            n272 = local write "M-"(w1059) -> ()
            n273 = local write "G+"(w1061) -> ()
            n274 = local write "Right+"(w1057) -> ()
            n275 = local write "Right-"(w1054) -> ()
            n276 = local write "Left+"(w1055) -> ()
            n277 = local write "Left-"(w1056) -> ()
            n278 = local write "G-"(w1062) -> ()
            n279 = local write "M+"(w1060) -> ()
          }
          frame "_Timer" {
            n280 = Wait (ms)(milliseconds to wait="_Timer") -> ()  [unwired: 1 out]
          }
          frame "Setup manipulator" {
            n281 = case shown="\"Release\"" "Manip state" {
              tunnel: ["G_UB_Align" w1083 w1085] -> w1072
              tunnel: ["M_UB_Align" w1084 w1085] -> w1073
              frame "Align", Default {
              }
              frame "Grab" {
                n282 = local read "M_UB_grab"() -> (w1084:i32)
                n283 = local read "G_UB_grab"() -> (w1083:i32)
              }
              frame "Release" {
                w1085 = 0
              }
            }
            n284 = call "Setup manipulator (SubVI).vi"("Release?"=FALSE, "G_upper bound"=w1072, "M_lower bound"=w1073, "error in (no error)"=w1076, "M_Encoder Ref In"=w1078, "G_Encoder Ref In"=w1077) -> ("error out"=w1075:errorcluster)  [unwired: 9 in]
          }
          frame "(auto) Count balls" {
            n285 = local read "Circles Calibrated (Shape Detection 1)"() -> (w1088:T3)
            n286 = call "(auto) Count balls (SubVI).vi"("Circles Calibrated (Shape Detection 1)"=w1088) -> ("balls counter"=w1089:i32)  [unwired: 10 in]
            "(auto) balls counter" <- w1089
            n287 = call "(auto) Skip same balls(SubVI).vi"("Circles Calibrated (Shape Detection 1)"=w1088, "balls counter"=w1089) -> ("balls coutnter Out"=w1086:i32, "arrOut"=→"balls to analyze":i32[])  [unwired: 8 in]
            n288 = local write "(auto) balls counter"(w1086) -> ()
          }
          frame "(auto) Analyze balls" {
            n289 = local read "(auto) balls counter"() -> (w1094:i32)
            n290 = Greater Than 0?(x=w1094) -> (x > 0?=w1095:bool)
            n291 = case shown="True" w1095 {
              tunnel: w1098 -> [_ w1107]
              tunnel: w1097 -> [w1102 w1106]
              tunnel: [w1102 w1105] -> w1096
              frame False {
              }
              frame True {
                n292 = flat-sequence {
                  tunnel: [w1109] -> w1104
                  tunnel: w1107 -> [w1123]
                  tunnel: w1106 -> [w1122]
                  tunnel: [w1121] -> w1105
                  tunnel: w1104 -> [w1119]
                  tunnel: [w1119] -> w1103
                  tunnel: w1103 -> [w1125]
                  frame #0 {
                    n293 = local read "Circles Calibrated (Shape Detection 1)"() -> (w1114:T3)
                    n294 = local read "balls to analyze"() -> (w1110:i32[])
                    n295 = local read "(auto) balls counter"() -> (w1109:i32)
                    n296 = Index Array(array=w1110, index=w1109) -> (element=w1108:i32)
                    n297 = Index Array(array=w1114, index=w1108) -> (element=w1118:T35)
                    n298 = Unbundle By Name(w1118) -> ("Position"=w1117:cluster{"X":sgl, "Y":sgl}, "Radius"=w1111:dbl)
                    n299 = Unbundle(w1117) -> ("X"=w1116:sgl, "Y"=w1115:sgl)
                    n300 = To Double Precision Float(number=w1116) -> (double precision float=w1113:dbl)
                    n301 = To Double Precision Float(number=w1115) -> (double precision float=w1112:dbl)
                    n302 = local write "CircleRadius"(w1111) -> ()
                    n303 = local write "curX"(w1113) -> ()
                    n304 = local write "curY"(w1112) -> ()
                  }
                  frame #1 {
                    w1120 = T33 [enum."(ball) Calculate ROI", enum."(ball) Analyze color", enum."(image) show", enum."Wait for button", enum."(auto) Analyze balls"] items=["(qsm) schedule", "(qsm) initialize", "(qsm) release", "(qsm) clean up", "(qsm) shutdown", "(myRIO) initialize", "(myRIO) clean up", "(myRIO) update ports", "Setup get", "(image) get", "(image) show", "(ball) Shape detection", "(ball) Calc ball indx", "(ball) Calculate ROI", "(ball) Analyze color", "(ball) Align", "(ball) Wait", "(ball) Grab", "(pattern) Find Square", "(pattern) Calculate ROI", "(pattern) Calc pattern indx", "Compare", "(pattern) Analyze pattern", "(pattern) Align", "(pattern) Wait", "(pattern) states control", "navx", "stop motors", "(joystick) Joystick control", "_Timer", "Setup manipulator", "(auto) Count balls", "(auto) Analyze balls", "(auto) Dot Controller", "Wait for button"] ("task")
                    n305 = call "enqueue_states.vi"("task"=w1120, "error in"=w1122, "queue in"=w1123) -> ("error out"=w1121:errorcluster)  [unwired: 6 in, 1 out]
                  }
                  frame #2 {
                    n306 = Decrement(x=w1125) -> (x-1=w1124:i32)
                    n307 = local write "(auto) balls counter"(w1124) -> ()
                    n308 = local write "Ball number"(w1124) -> ()
                  }
                }
              }
            }
          }
          frame "(auto) Dot Controller" {
            # "here we should get and save: angle, L/R/M/G_enc's"
            # "here we should decide which of (auto) States we must use (DON'T USE 0)"
            n309 = flat-sequence {
              tunnel: w1138 -> [w1159]
              tunnel: w1137 -> [w1158]
              tunnel: w1136 -> [w1145]
              tunnel: w1135 -> [w1144]
              tunnel: w1134 -> [w1143]
              tunnel: w1133 -> [w1142]
              tunnel: [w1141] -> w1131
              tunnel: [w1157] -> w1129
              tunnel: w1129 -> [w1166]
              tunnel: [w1166] -> w1128
              tunnel: [w1169] -> w1126
              tunnel: w1128 -> [w1169]
              tunnel: [w1167] -> w1127
              frame #0 {
                n310 = local read "Angles"() -> (w1155:dbl[])
                n311 = local read "Left_enc"() -> (w1154:i32[])
                n312 = local read "Right_enc"() -> (w1153:i32[])
                n313 = local read "M_enc"() -> (w1152:i32[])
                n314 = local read "G_enc"() -> (w1151:i32[])
                n315 = Increment(x="CurDot") -> (x+1=w1156:T2)
                n316 = local write "CurDot"(w1156) -> ()
                n317 = call "(auto) SAVE.vi"("I2C Ref Out in"=w1159, "CurDot"=w1156, "Angles"=w1155, "Left_enc"=w1154, "Right_enc"=w1153, "M_enc"=w1152, "G_enc"=w1151, "error in (no error)"=w1158, "L_enc In"=w1145, "R_enc In"=w1144, "M_enc In"=w1143, "G_enc In"=w1142) -> ("I2C Ref Out out"=w1157:T22, "Angles out"=w1150:dbl[], "Left_enc out"=w1149:i32[], "Right_enc out"=w1148:i32[], "M_enc out"=w1147:i32[], "G_enc out"=w1146:i32[], "error out"=w1141:errorcluster)  [unwired: 9 in]
                n318 = local write "Angles"(w1150) -> ()
                n319 = local write "Left_enc"(w1149) -> ()
                n320 = local write "Right_enc"(w1148) -> ()
                n321 = local write "M_enc"(w1147) -> ()
                n322 = local write "G_enc"(w1146) -> ()
              }
              frame #1 {
                n323 = local read "States in total"() -> (w1165:i32)
                n324 = local read "Dots of States"() -> (w1163:i32[][])
                n325 = local read "Dots in total"() -> (w1162:i32)
                n326 = local read "CurDot"() -> (w1164:T2)
                n327 = call "(auto) Get State (SubVI).vi"("Dots in total"=w1162, "States in total"=w1165, "CurDot"=w1164, "Dots of States"=w1163) -> ("(auto) States"=w1161:T2)  [unwired: 7 in]
                n328 = local write "(auto) States"(w1161) -> ()
              }
              frame #2 {
                n329 = case shown="\"1\"" "(auto) States" {
                  tunnel: [w1170 w1171 w1172 w1173 w1174 w1175 w1176 w1177 w1178 w1179 w1180] -> w1167
                  frame "0", Default {
                    w1170 = T33 [enum."(qsm) shutdown"] items=["(qsm) schedule", "(qsm) initialize", "(qsm) release", "(qsm) clean up", "(qsm) shutdown", "(myRIO) initialize", "(myRIO) clean up", "(myRIO) update ports", "Setup get", "(image) get", "(image) show", "(ball) Shape detection", "(ball) Calc ball indx", "(ball) Calculate ROI", "(ball) Analyze color", "(ball) Align", "(ball) Wait", "(ball) Grab", "(pattern) Find Square", "(pattern) Calculate ROI", "(pattern) Calc pattern indx", "Compare", "(pattern) Analyze pattern", "(pattern) Align", "(pattern) Wait", "(pattern) states control", "navx", "stop motors", "(joystick) Joystick control", "_Timer", "Setup manipulator", "(auto) Count balls", "(auto) Analyze balls", "(auto) Dot Controller", "Wait for button"] ("task")
                    # "DON'T USE 0"
                  }
                  frame "1" {
                    w1171 = T33 [enum."(qsm) initialize"] items=["(qsm) schedule", "(qsm) initialize", "(qsm) release", "(qsm) clean up", "(qsm) shutdown", "(myRIO) initialize", "(myRIO) clean up", "(myRIO) update ports", "Setup get", "(image) get", "(image) show", "(ball) Shape detection", "(ball) Calc ball indx", "(ball) Calculate ROI", "(ball) Analyze color", "(ball) Align", "(ball) Wait", "(ball) Grab", "(pattern) Find Square", "(pattern) Calculate ROI", "(pattern) Calc pattern indx", "Compare", "(pattern) Analyze pattern", "(pattern) Align", "(pattern) Wait", "(pattern) states control", "navx", "stop motors", "(joystick) Joystick control", "_Timer", "Setup manipulator", "(auto) Count balls", "(auto) Analyze balls", "(auto) Dot Controller", "Wait for button"] ("task")
                  }
                  frame "2" {
                    w1172 = T33 [enum."(qsm) initialize"] items=["(qsm) schedule", "(qsm) initialize", "(qsm) release", "(qsm) clean up", "(qsm) shutdown", "(myRIO) initialize", "(myRIO) clean up", "(myRIO) update ports", "Setup get", "(image) get", "(image) show", "(ball) Shape detection", "(ball) Calc ball indx", "(ball) Calculate ROI", "(ball) Analyze color", "(ball) Align", "(ball) Wait", "(ball) Grab", "(pattern) Find Square", "(pattern) Calculate ROI", "(pattern) Calc pattern indx", "Compare", "(pattern) Analyze pattern", "(pattern) Align", "(pattern) Wait", "(pattern) states control", "navx", "stop motors", "(joystick) Joystick control", "_Timer", "Setup manipulator", "(auto) Count balls", "(auto) Analyze balls", "(auto) Dot Controller", "Wait for button"] ("task")
                  }
                  frame "3" {
                    w1173 = T33 [enum."(qsm) initialize"] items=["(qsm) schedule", "(qsm) initialize", "(qsm) release", "(qsm) clean up", "(qsm) shutdown", "(myRIO) initialize", "(myRIO) clean up", "(myRIO) update ports", "Setup get", "(image) get", "(image) show", "(ball) Shape detection", "(ball) Calc ball indx", "(ball) Calculate ROI", "(ball) Analyze color", "(ball) Align", "(ball) Wait", "(ball) Grab", "(pattern) Find Square", "(pattern) Calculate ROI", "(pattern) Calc pattern indx", "Compare", "(pattern) Analyze pattern", "(pattern) Align", "(pattern) Wait", "(pattern) states control", "navx", "stop motors", "(joystick) Joystick control", "_Timer", "Setup manipulator", "(auto) Count balls", "(auto) Analyze balls", "(auto) Dot Controller", "Wait for button"] ("task")
                  }
                  frame "4" {
                    w1174 = T33 [enum."(qsm) initialize"] items=["(qsm) schedule", "(qsm) initialize", "(qsm) release", "(qsm) clean up", "(qsm) shutdown", "(myRIO) initialize", "(myRIO) clean up", "(myRIO) update ports", "Setup get", "(image) get", "(image) show", "(ball) Shape detection", "(ball) Calc ball indx", "(ball) Calculate ROI", "(ball) Analyze color", "(ball) Align", "(ball) Wait", "(ball) Grab", "(pattern) Find Square", "(pattern) Calculate ROI", "(pattern) Calc pattern indx", "Compare", "(pattern) Analyze pattern", "(pattern) Align", "(pattern) Wait", "(pattern) states control", "navx", "stop motors", "(joystick) Joystick control", "_Timer", "Setup manipulator", "(auto) Count balls", "(auto) Analyze balls", "(auto) Dot Controller", "Wait for button"] ("task")
                  }
                  frame "5" {
                    w1175 = T33 [enum."(qsm) initialize"] items=["(qsm) schedule", "(qsm) initialize", "(qsm) release", "(qsm) clean up", "(qsm) shutdown", "(myRIO) initialize", "(myRIO) clean up", "(myRIO) update ports", "Setup get", "(image) get", "(image) show", "(ball) Shape detection", "(ball) Calc ball indx", "(ball) Calculate ROI", "(ball) Analyze color", "(ball) Align", "(ball) Wait", "(ball) Grab", "(pattern) Find Square", "(pattern) Calculate ROI", "(pattern) Calc pattern indx", "Compare", "(pattern) Analyze pattern", "(pattern) Align", "(pattern) Wait", "(pattern) states control", "navx", "stop motors", "(joystick) Joystick control", "_Timer", "Setup manipulator", "(auto) Count balls", "(auto) Analyze balls", "(auto) Dot Controller", "Wait for button"] ("task")
                  }
                  frame "6" {
                    w1176 = T33 [enum."(qsm) initialize"] items=["(qsm) schedule", "(qsm) initialize", "(qsm) release", "(qsm) clean up", "(qsm) shutdown", "(myRIO) initialize", "(myRIO) clean up", "(myRIO) update ports", "Setup get", "(image) get", "(image) show", "(ball) Shape detection", "(ball) Calc ball indx", "(ball) Calculate ROI", "(ball) Analyze color", "(ball) Align", "(ball) Wait", "(ball) Grab", "(pattern) Find Square", "(pattern) Calculate ROI", "(pattern) Calc pattern indx", "Compare", "(pattern) Analyze pattern", "(pattern) Align", "(pattern) Wait", "(pattern) states control", "navx", "stop motors", "(joystick) Joystick control", "_Timer", "Setup manipulator", "(auto) Count balls", "(auto) Analyze balls", "(auto) Dot Controller", "Wait for button"] ("task")
                  }
                  frame "7" {
                    w1177 = T33 [enum."(qsm) initialize"] items=["(qsm) schedule", "(qsm) initialize", "(qsm) release", "(qsm) clean up", "(qsm) shutdown", "(myRIO) initialize", "(myRIO) clean up", "(myRIO) update ports", "Setup get", "(image) get", "(image) show", "(ball) Shape detection", "(ball) Calc ball indx", "(ball) Calculate ROI", "(ball) Analyze color", "(ball) Align", "(ball) Wait", "(ball) Grab", "(pattern) Find Square", "(pattern) Calculate ROI", "(pattern) Calc pattern indx", "Compare", "(pattern) Analyze pattern", "(pattern) Align", "(pattern) Wait", "(pattern) states control", "navx", "stop motors", "(joystick) Joystick control", "_Timer", "Setup manipulator", "(auto) Count balls", "(auto) Analyze balls", "(auto) Dot Controller", "Wait for button"] ("task")
                  }
                  frame "8" {
                    w1178 = T33 [enum."(qsm) initialize"] items=["(qsm) schedule", "(qsm) initialize", "(qsm) release", "(qsm) clean up", "(qsm) shutdown", "(myRIO) initialize", "(myRIO) clean up", "(myRIO) update ports", "Setup get", "(image) get", "(image) show", "(ball) Shape detection", "(ball) Calc ball indx", "(ball) Calculate ROI", "(ball) Analyze color", "(ball) Align", "(ball) Wait", "(ball) Grab", "(pattern) Find Square", "(pattern) Calculate ROI", "(pattern) Calc pattern indx", "Compare", "(pattern) Analyze pattern", "(pattern) Align", "(pattern) Wait", "(pattern) states control", "navx", "stop motors", "(joystick) Joystick control", "_Timer", "Setup manipulator", "(auto) Count balls", "(auto) Analyze balls", "(auto) Dot Controller", "Wait for button"] ("task")
                  }
                  frame "9" {
                    w1179 = T33 [enum."(qsm) initialize"] items=["(qsm) schedule", "(qsm) initialize", "(qsm) release", "(qsm) clean up", "(qsm) shutdown", "(myRIO) initialize", "(myRIO) clean up", "(myRIO) update ports", "Setup get", "(image) get", "(image) show", "(ball) Shape detection", "(ball) Calc ball indx", "(ball) Calculate ROI", "(ball) Analyze color", "(ball) Align", "(ball) Wait", "(ball) Grab", "(pattern) Find Square", "(pattern) Calculate ROI", "(pattern) Calc pattern indx", "Compare", "(pattern) Analyze pattern", "(pattern) Align", "(pattern) Wait", "(pattern) states control", "navx", "stop motors", "(joystick) Joystick control", "_Timer", "Setup manipulator", "(auto) Count balls", "(auto) Analyze balls", "(auto) Dot Controller", "Wait for button"] ("task")
                  }
                  frame "10" {
                    w1180 = T33 [enum."(qsm) initialize"] items=["(qsm) schedule", "(qsm) initialize", "(qsm) release", "(qsm) clean up", "(qsm) shutdown", "(myRIO) initialize", "(myRIO) clean up", "(myRIO) update ports", "Setup get", "(image) get", "(image) show", "(ball) Shape detection", "(ball) Calc ball indx", "(ball) Calculate ROI", "(ball) Analyze color", "(ball) Align", "(ball) Wait", "(ball) Grab", "(pattern) Find Square", "(pattern) Calculate ROI", "(pattern) Calc pattern indx", "Compare", "(pattern) Analyze pattern", "(pattern) Align", "(pattern) Wait", "(pattern) states control", "navx", "stop motors", "(joystick) Joystick control", "_Timer", "Setup manipulator", "(auto) Count balls", "(auto) Analyze balls", "(auto) Dot Controller", "Wait for button"] ("task")
                  }
                }
              }
            }
            n330 = call "enqueue_states.vi"("task"=w1127, "error in"=w1131, "queue in"=w1132) -> ("error out"=w1130:errorcluster)  [unwired: 6 in, 1 out]
          }
          frame "Wait for button" {
            n331 = while {
              stop <- w1188 stop-if-true
              n332 = local read "Stop"() -> (w1190:bool)
              n333 = xnode "Button 2"() -> ("Value"=w1186:bool)  [unwired: 1 in, 1 out]
              n334 = Or(x="Next step", y=w1190) -> (x .or. y?=w1187:bool)
              n335 = Or(x=w1187, y=w1186) -> (x .or. y?=w1188:bool)
            }
            n336 = local write "Next step"(FALSE ("Look at ball")) -> ()
          }
        }
        n337 = Merge Errors(w183, w182) -> (w170:errorcluster)
        n338 = local read "ball match"() -> (w143:bool)
        n339 = local read "pattern match"() -> (w141:bool)
        n340 = Or(x=w143, y="ball = pattern?") -> (x .or. y?=w144:bool)
        n341 = Or(x=w144, y=w141) -> (x .or. y?=w142:bool)
        n342 = xnode "LED"("LED0"=w142, "LED1"=w142, "LED2"=w142, "LED3"=w142, "error in (no error)"=w170) -> ("error out"=w169:errorcluster)
        n343 = Unbundle By Name(w165) -> ("Pattern classes"=w168:i32[], "Color classes"=w160:i32[])
        "Color classes" <- w160
        "Pattern classes" <- w168
        n344 = Merge Errors(w161, w169) -> (w185:errorcluster)
        n345 = local read "Number of Matches (Shape Detection 1)"() -> (w167:i32)
        n346 = local read "Ball number"() -> (w159:i32)
        n347 = Index Array(array=w168) -> (element=w145:i32)  [unwired: 1 in]
        n348 = Index Array(array=w160, index=w159) -> (element=w146:i32)
        n349 = Equal?(x=w146, y="1") -> (x = y?=→"1":bool)
        n350 = Equal?(x=w146, y="2") -> (x = y?=→"2":bool)
        n351 = Equal?(x=w146, y="3") -> (x = y?=→"3":bool)
        n352 = Equal?(x=w146, y="4") -> (x = y?=→"4":bool)
        n353 = Equal?(x=w146, y="5") -> (x = y?=→"5":bool)
        n354 = Equal?(x=w145, y=w146) -> (x = y?=w162:bool)
        n355 = local write "ball = pattern?"(w162) -> ()
        n356 = Greater Than 0?(x=w167) -> (x > 0?=w166:bool)
        n357 = case shown="True" w166 {
          tunnel: [w231 w237] -> w164
          tunnel: w165 -> [w230 w237]
          frame False {
            n358 = Unbundle By Name(w230) -> ("Color classes"=w227:i32[])
            n359 = for {
              N: 5 -> [w235]
              tunnel: [w236] -> w229
              tunnel: w227 -> [w233]
              n360 = Decrement(x=w235) -> (x-1=w234:i32)
              n361 = Replace Array Subset(array=w233, new element=20, index=w234) -> (w236:i32[])
            }
            n362 = Bundle By Name(cluster=w230, "Color classes"=w229) -> (w231:T10)
          }
          frame True {
          }
        }
      }
    }
    frame #1 {
      w1237 = 0 ("G_upper bound")
      w1248 = 1 ("Ball index")
      w1239 = FALSE ("X is in range")
      n363 = disable-structure shown="Disabled" {
        disable-tunnel: w1244 -> [w1252 _]
        disable-tunnel: [w1251 _] -> w1243
        disable-tunnel: w1238 -> [w1250 _]
        frame Disabled {
          n364 = call <vilib>:"Close.vi"("error in (no error)"=w1250, "I2C Ref In"=w1252) -> ("error out"=w1251:errorcluster)  [unwired: 9 in]
        }
        frame Enabled {
        }
      }
      n365 = call "Setup manipulator (SubVI).vi"("Release?"=TRUE, "G_upper bound"=w1237, "M_lower bound"=w1237, "error in (no error)"=w1238, "M_Encoder Ref In"=w1234, "G_Encoder Ref In"=w1233) -> ("error out"=w1230:errorcluster)  [unwired: 9 in]
      n366 = call <vilib>:"Close.vi"("error in (no error)"=w1238, "PWM Ref In"=w1236) -> ("error out"=w1245:errorcluster)  [unwired: 9 in]
      n367 = call <vilib>:"Close.vi"("error in (no error)"=w1238, "PWM Ref In"=w1235) -> ("error out"=w1246:errorcluster)  [unwired: 9 in]
      n368 = call <vilib>:"Close.vi"("error in (no error)"=w1230, "Encoder Ref In"=w1234) -> ("error out"=w1240:errorcluster)  [unwired: 9 in]
      n369 = call <vilib>:"Close.vi"("error in (no error)"=w1230, "Encoder Ref In"=w1233) -> ("error out"=w1241:errorcluster)  [unwired: 9 in]
      n370 = call <vilib>:"Close.vi"("error in (no error)"=w1230, "Encoder Ref In"=w1228) -> ("error out"=w1227:errorcluster)  [unwired: 9 in]
      n371 = call <vilib>:"Close.vi"("error in (no error)"=w1230, "Encoder Ref In"=w1229) -> ("error out"=w1226:errorcluster)  [unwired: 9 in]
      n372 = Merge Errors(w1243, w1238, w1245, w1246, w1240, w1241, w1227, w1226) -> (w1247:errorcluster)
      n373 = local write "(auto) balls counter"(0 ("(auto) balls counter")) -> ()
      n374 = local write "Ball number"(w1248) -> ()
      n375 = local write "pattern number"(w1248) -> ()
      n376 = call <vilib>:"Simple Error Handler.vi"("error in (no error)"=w1247) -> ("error out"=w1249:errorcluster)  [unwired: 4 in, 4 out]
      "error out" <- w1249
      n377 = local write "ball = pattern?"(w1239) -> ()
      n378 = local write "X is in range"(w1239) -> ()
      n379 = local write "Y is in range"(w1239) -> ()
      n380 = local write "Next step"(w1239) -> ()
      n381 = shared-variable "myRIO-1900\\vars.lvlib\\def Z"(ext -800.0 ("def Z")) -> ()  [unwired: 1 in, 1 out]
      n382 = local write "Right+"(w1239) -> ()
      n383 = local write "Right-"(w1239) -> ()
      n384 = local write "rotate"(w1239) -> ()
      n385 = local write "Left+"(w1239) -> ()
      n386 = local write "Left-"(w1239) -> ()
      n387 = local write "Stop"(w1239) -> ()
      n388 = local write "M+"(w1239) -> ()
      n389 = local write "G+"(w1239) -> ()
      n390 = local write "M-"(w1239) -> ()
      n391 = local write "G-"(w1239) -> ()
    }
  }
  n392 = call <vilib>:"Reset myRIO.vi"("error in (no error)"=w52) -> ()  [unwired: 10 in, 1 out]
